vi "Roper DOE Gas Volume Consumed.vi"() -> ()   [LabVIEW 2012]
uses:
  <vilib>/DAQmx/read.llb/DAQmx Read (Analog 1D DBL NChan 1Samp).vi
  <vilib>/DAQmx/miscellaneous.llb/DAQmx Fill In Error Info.vi
panel:
  out "LP":bool
  out "NG":bool
  out "25%Sum":dbl
  out "MaxRateSum":dbl
  out "25%RateTime":dbl
  out "MaxRateTime":dbl
  out "CurrentState":string
  in  "Data Sampling Rate (s)":dbl=1.0
  out "Second":dbl format="%#.0f"
  out "Minute":dbl format="%#.0f"
  out "25PercentInRange":bool
  out "25PercentRate":bool
  out "MaxRateState":bool
  out "25% Rate Run Average":dbl format="%#.0f"
  out "Target 25% Average":dbl format="%#.0f"
  out "Max Rate Run Avg.":dbl format="%#.0f"
  out "HV":dbl
  out "CF HR":dbl
  out "Meter SLPM":dbl
  out "Sum Time":dbl
  in  "Gas Type":string
  out "Current Meter":dbl
  in  "Reset":bool
  out "Seconds":dbl format="%#.0f"
  out "Minutes":dbl format="%#.0f"
  out "Cubic Ft. Flowed":dbl format="%#.3f"
  out "Signal 2":bool
  out "Reference6":dbl
  out "Reference5":dbl
  out "Reference4":dbl
  out "Reference3":dbl
  out "Reference2":dbl
  out "Reference1":dbl
  in  "HeatingValueLP":dbl=2450.0 min=2400.0 max=2600.0 step=1.0
  out "Output 6":dbl min=0.0 max=5.0 step=0.01
  out "Output 5":dbl min=0.0 max=5.0 step=0.01
  out "Output 4":dbl min=0.0 max=5.0 step=0.01
  out "Output 3":dbl min=0.0 max=5.0 step=0.01
  out "Output 2":dbl min=0.0 max=5.0 step=0.01
  out "Output 1":dbl min=0.0 max=5.0 step=0.01
  in  "HeatingValueNG":dbl=990.0 min=950.0 max=1050.0 step=1.0
  out "Flow Rate":dbl format="%#.0f"
  # "Instant Flow Rate (BTU/hr)"
  # "Signal"
  # "Dry Heating Value"
  # "Elapsed Time"
  # ":"
  # "In Range"
  # "25% Rate Countdown Timer"
  # ":"
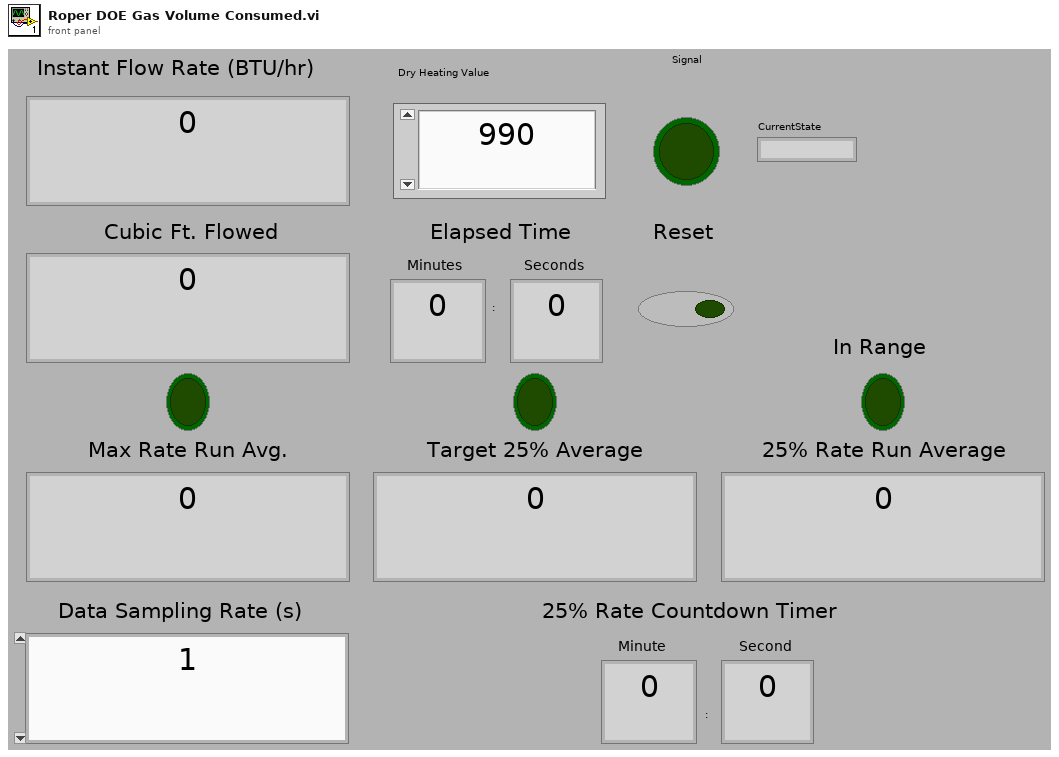
[diagram p1: front panel]
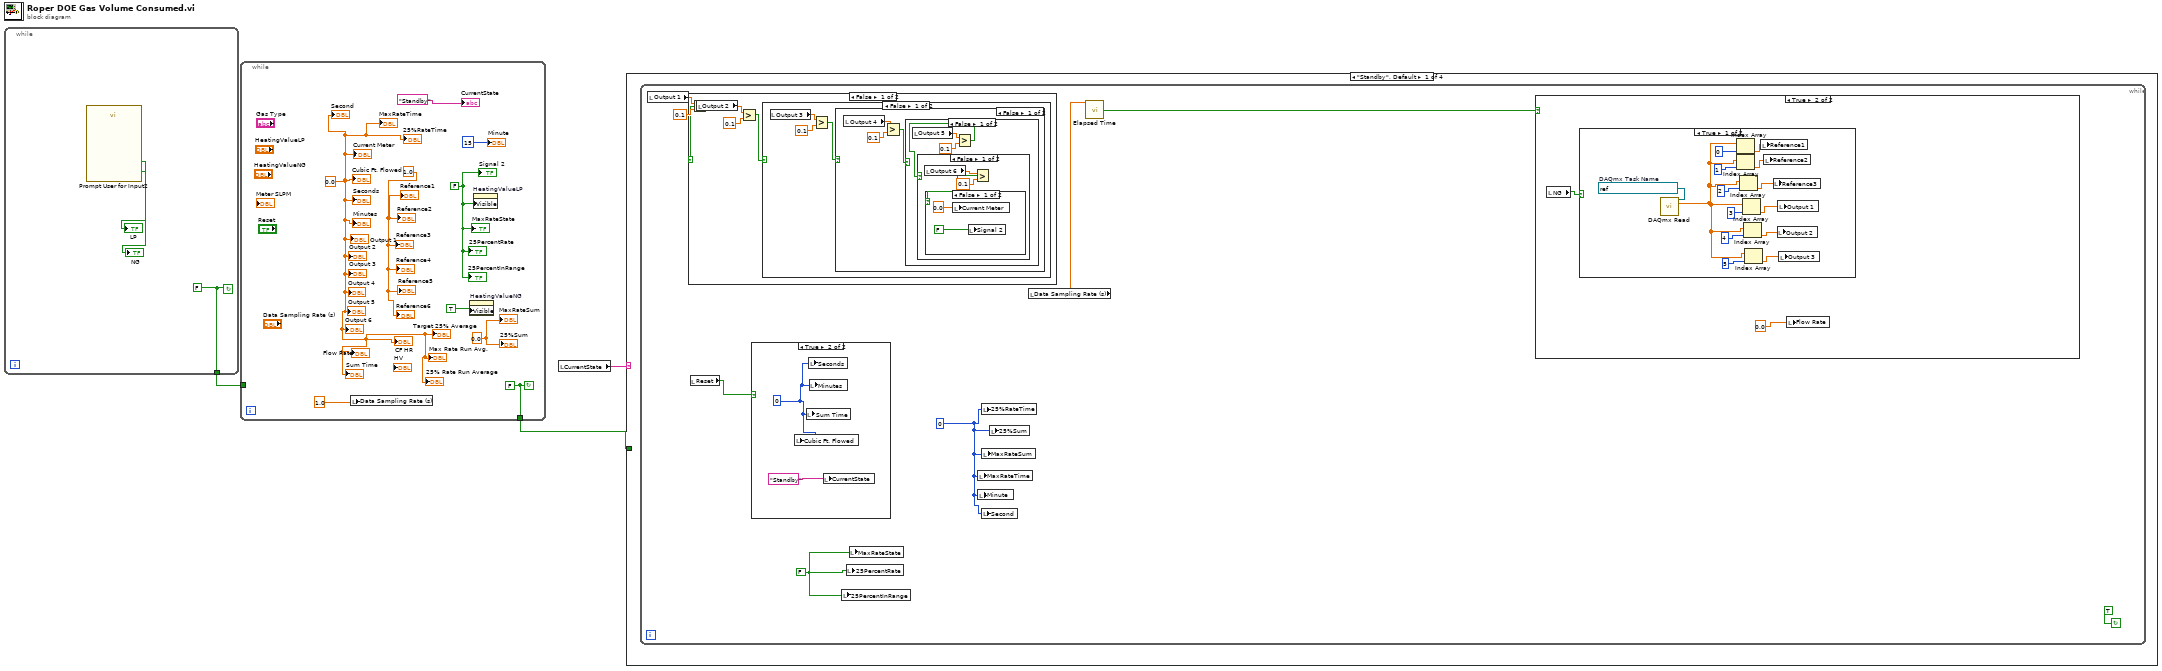
[diagram p0: block diagram]
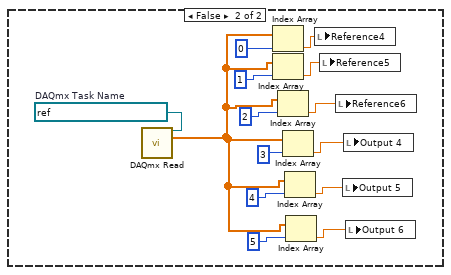
[diagram p3: hidden frame]
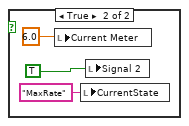
[diagram p4: hidden frame]
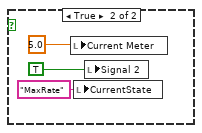
[diagram p5: hidden frame]
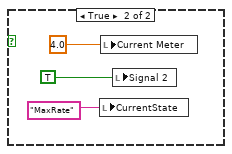
[diagram p6: hidden frame]
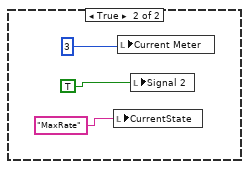
[diagram p7: hidden frame]
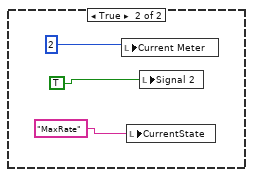
[diagram p8: hidden frame]
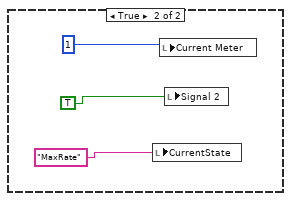
[diagram p9: hidden frame]
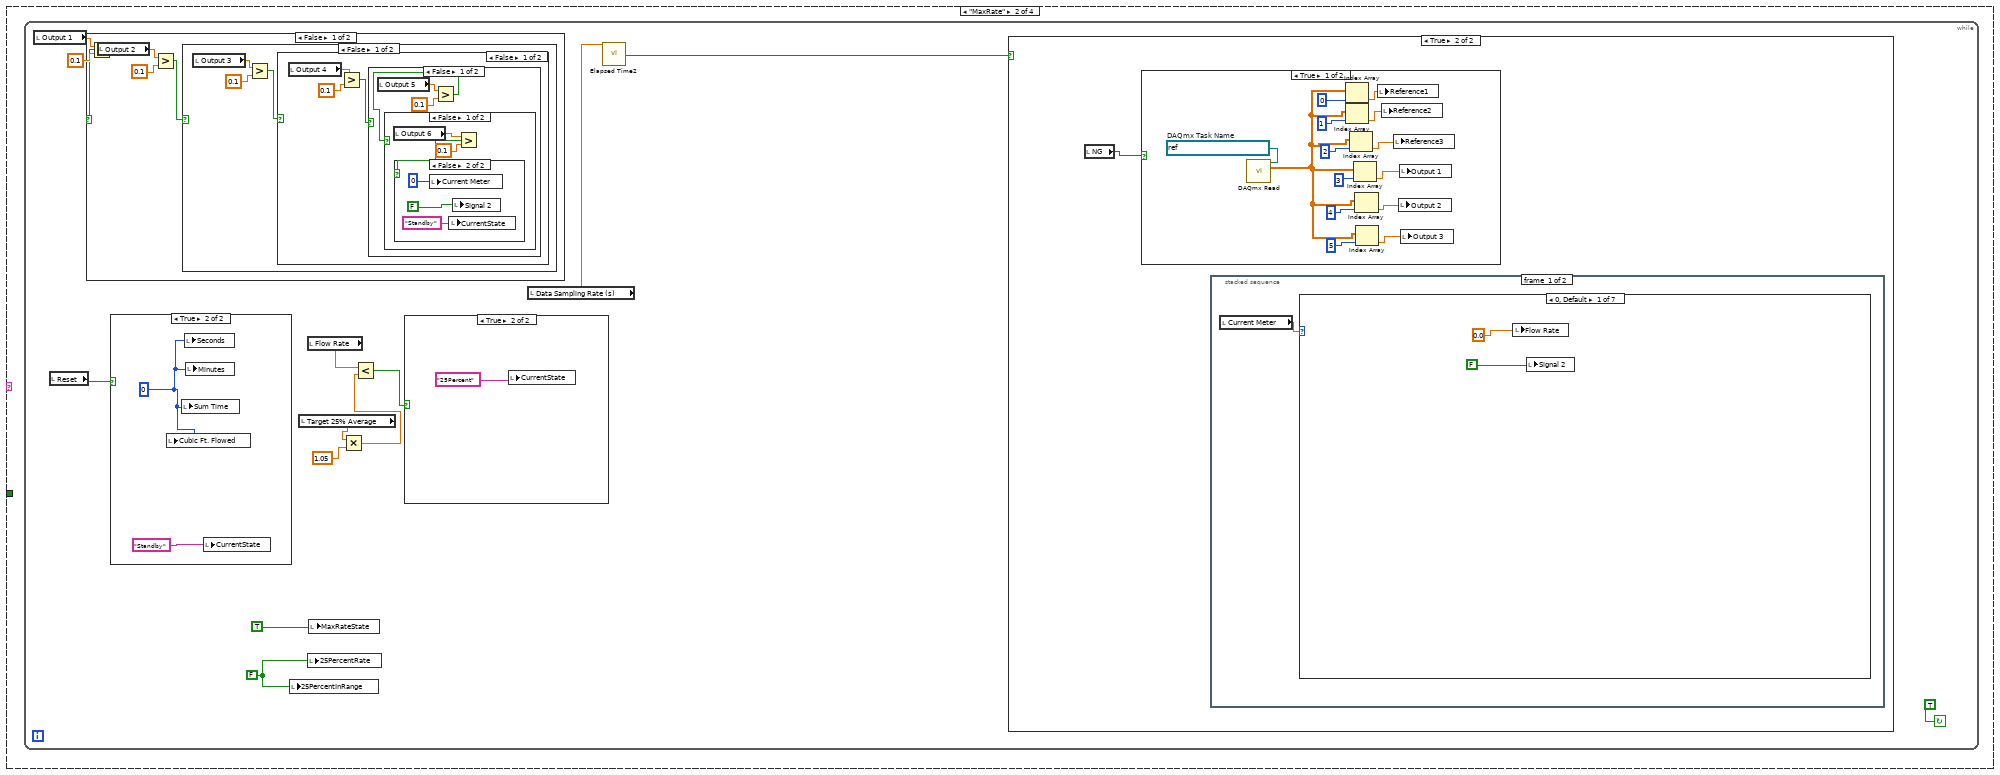
[diagram p11: hidden frame]
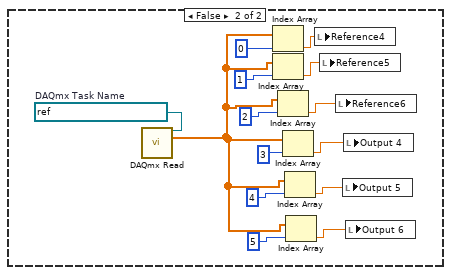
[diagram p14: hidden frame]
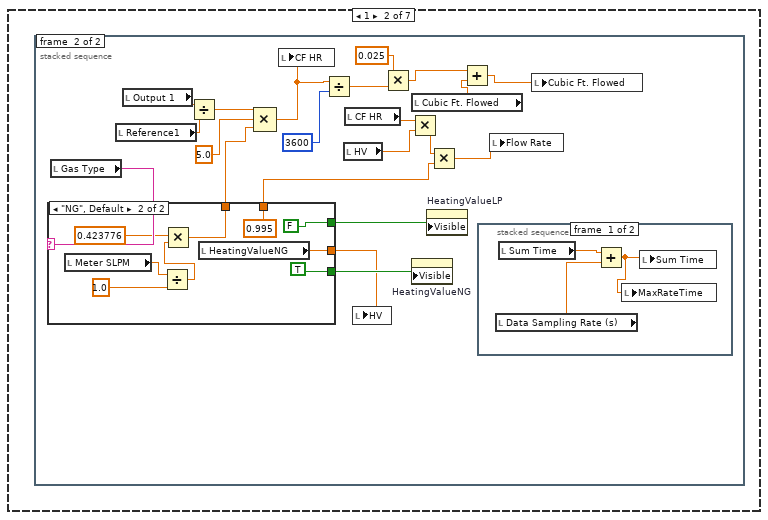
[diagram p15: hidden frame]
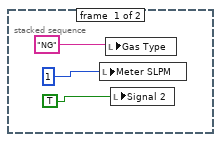
[diagram p16: hidden frame]
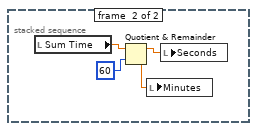
[diagram p17: hidden frame]
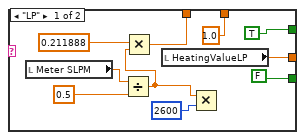
[diagram p18: hidden frame]
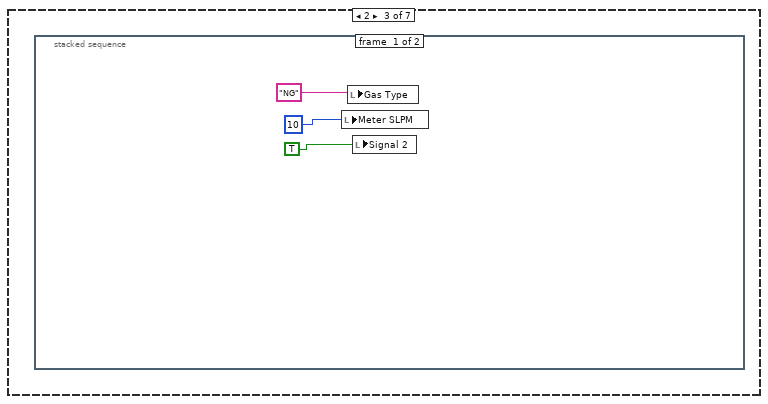
[diagram p19: hidden frame]
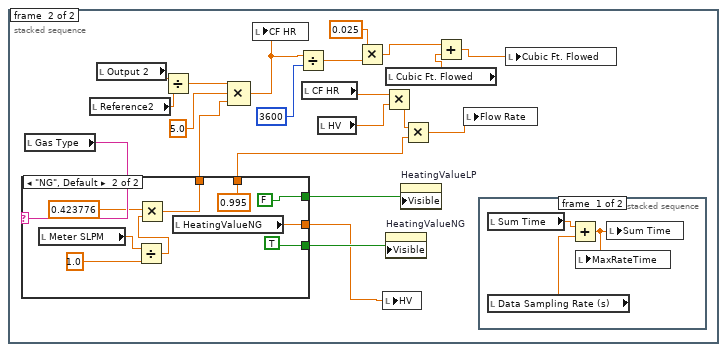
[diagram p20: hidden frame]
diagram:
  n1 = while {
    tunnel: [w6] -> w2
    stop <- w6 continue-if-true
    w6 = FALSE
    n2 = call "Prompt User for Input2"() -> ("LP"=→"LP":bool, "NG"=→"NG":bool)  [unwired: 16 in, 2 out]
  }
  n3 = while {
    tunnel: w2 -> [_]
    tunnel: [w9] -> w1
    stop <- w9 continue-if-true
    w10 = 0.0
    w13 = FALSE
    w15 = 1.0
    w8 = 0.0
    w9 = FALSE
    n4 = local write "Data Sampling Rate (s)"(1.0) -> ()
    n5 = property on="HeatingValueNG" class="DigNum (strict)"("Visible"=TRUE) -> ()  [unwired: 2 in, 2 out]
    n6 = property on="HeatingValueLP" class="DigNum (strict)"("Visible"=w13) -> ()  [unwired: 2 in, 2 out]
    "Output 1" <- w8
    "Output 2" <- w8
    "Output 3" <- w8
    "Output 4" <- w8
    "Output 5" <- w8
    "Output 6" <- w8
    "Reference1" <- w15
    "Reference2" <- w15
    "Reference3" <- w15
    "Reference4" <- w15
    "Reference5" <- w15
    "Reference6" <- w15
    "Flow Rate" <- w8
    "Signal 2" <- w13
    "Cubic Ft. Flowed" <- w8
    "Minutes" <- w8
    "Seconds" <- w8
    "Current Meter" <- w8
    "Sum Time" <- w8
    "CF HR" <- w8
    "Max Rate Run Avg." <- w8
    "Target 25% Average" <- w8
    "25% Rate Run Average" <- w8
    "MaxRateState" <- w13
    "25PercentRate" <- w13
    "25PercentInRange" <- w13
    "Minute" <- 15
    "Second" <- w8
    "CurrentState" <- "Standby"
    "25%RateTime" <- w8
    "MaxRateTime" <- w8
    "25%Sum" <- w10
    "MaxRateSum" <- w10
  }
  n7 = local read "CurrentState"() -> (w3:string)
  n8 = case shown="\"Standby\", Default" w3 {
    tunnel: w1 -> [_ _ _ _]
    frame "Standby", Default {
      n9 = while {
        stop <- TRUE continue-if-true
        w16 = 0
        w17 = FALSE
        n10 = local read "Output 1"() -> (w21:dbl)
        n11 = local read "Reset"() -> (w23:bool)
        n12 = Greater?(x=w21, y=0.1) -> (0:w20:bool)
        n13 = case shown="False" w20 {
          frame False {
            n14 = local read "Output 2"() -> (w56:dbl)
            n15 = Greater?(x=w56, y=0.1) -> (0:w55:bool)
            n16 = case shown="False" w55 {
              frame False {
                n17 = local read "Output 3"() -> (w59:dbl)
                n18 = Greater?(x=w59, y=0.1) -> (0:w58:bool)
                n19 = case shown="False" w58 {
                  frame False {
                    n20 = local read "Output 4"() -> (w63:dbl)
                    n21 = Greater?(x=w63, y=0.1) -> (0:w61:bool)
                    n22 = case shown="False" w61 {
                      frame False {
                        n23 = local read "Output 5"() -> (w66:dbl)
                        n24 = Greater?(x=w66, y=0.1) -> (0:w64:bool)
                        n25 = case shown="False" w64 {
                          frame False {
                            n26 = local read "Output 6"() -> (w68:dbl)
                            n27 = Greater?(x=w68, y=0.1) -> (0:w67:bool)
                            n28 = case shown="False" w67 {
                              frame False {
                                n29 = local write "Current Meter"(0.0) -> ()
                                n30 = local write "Signal 2"(FALSE) -> ()
                              }
                              frame True {
                                n31 = local write "Current Meter"(6.0) -> ()
                                n32 = local write "CurrentState"("MaxRate") -> ()
                                n33 = local write "Signal 2"(TRUE) -> ()
                              }
                            }
                          }
                          frame True {
                            n34 = local write "Current Meter"(5.0) -> ()
                            n35 = local write "CurrentState"("MaxRate") -> ()
                            n36 = local write "Signal 2"(TRUE) -> ()
                          }
                        }
                      }
                      frame True {
                        n37 = local write "CurrentState"("MaxRate") -> ()
                        n38 = local write "Current Meter"(4.0) -> ()
                        n39 = local write "Signal 2"(TRUE) -> ()
                      }
                    }
                  }
                  frame True {
                    n40 = local write "CurrentState"("MaxRate") -> ()
                    n41 = local write "Current Meter"(3) -> ()
                    n42 = local write "Signal 2"(TRUE) -> ()
                  }
                }
              }
              frame True {
                n43 = local write "Current Meter"(2) -> ()
                n44 = local write "CurrentState"("MaxRate") -> ()
                n45 = local write "Signal 2"(TRUE) -> ()
              }
            }
          }
          frame True {
            n46 = local write "CurrentState"("MaxRate") -> ()
            n47 = local write "Current Meter"(1) -> ()
            n48 = local write "Signal 2"(TRUE) -> ()
          }
        }
        n49 = case shown="True" w23 {
          frame False {
          }
          frame True {
            w91 = 0
            n50 = local write "Cubic Ft. Flowed"(w91) -> ()
            n51 = local write "Sum Time"(w91) -> ()
            n52 = local write "Seconds"(w91) -> ()
            n53 = local write "Minutes"(w91) -> ()
            n54 = local write "CurrentState"("Standby") -> ()
          }
        }
        n55 = local write "25PercentInRange"(w17) -> ()
        n56 = local write "25PercentRate"(w17) -> ()
        n57 = local write "MaxRateState"(w17) -> ()
        n58 = local write "MaxRateTime"(w16) -> ()
        n59 = local write "Minute"(w16) -> ()
        n60 = local write "25%RateTime"(w16) -> ()
        n61 = local write "Second"(w16) -> ()
        n62 = local write "MaxRateSum"(w16) -> ()
        n63 = local write "25%Sum"(w16) -> ()
        n64 = local read "Data Sampling Rate (s)"() -> (w18:dbl)
        n65 = call "Elapsed Time"("Time Target (s)"=w18) -> ("Time has Elapsed"=w19:bool)  [unwired: 11 in, 7 out]
        n66 = case shown="True" w19 {
          frame False {
          }
          frame True {
            n67 = local read "NG"() -> (w25:bool)
            n68 = case shown="True" w25 {
              frame True {
                w40 = refnum<k21> "ReadNGFlowMeterIn"  # DAQmx Task Name
                n69 = call-poly <vilib>:"DAQmx Read.vi"("task/channels in"=w40) -> ("data"=w31:dbl[])  [unwired: 12 in, 2 out]
                n70 = Index Array(array=w31, index=0) -> (element=w36:dbl)
                n71 = Index Array(array=w31, index=1) -> (element=w37:dbl)
                n72 = Index Array(array=w31, index=2) -> (element=w30:dbl)
                n73 = Index Array(array=w31, index=3) -> (element=w29:dbl)
                n74 = Index Array(array=w31, index=4) -> (element=w28:dbl)
                n75 = Index Array(array=w31, index=5) -> (element=w27:dbl)
                n76 = local write "Reference1"(w36) -> ()
                n77 = local write "Reference2"(w37) -> ()
                n78 = local write "Reference3"(w30) -> ()
                n79 = local write "Output 2"(w28) -> ()
                n80 = local write "Output 1"(w29) -> ()
                n81 = local write "Output 3"(w27) -> ()
              }
              frame False {
                w54 = refnum<k21> "ReadLPFlowMeterIn"  # DAQmx Task Name
                n82 = call-poly <vilib>:"DAQmx Read.vi"("task/channels in"=w54) -> ("data"=w45:dbl[])  [unwired: 12 in, 2 out]
                n83 = Index Array(array=w45, index=0) -> (element=w50:dbl)
                n84 = Index Array(array=w45, index=1) -> (element=w51:dbl)
                n85 = Index Array(array=w45, index=2) -> (element=w44:dbl)
                n86 = Index Array(array=w45, index=3) -> (element=w43:dbl)
                n87 = Index Array(array=w45, index=4) -> (element=w42:dbl)
                n88 = Index Array(array=w45, index=5) -> (element=w41:dbl)
                n89 = local write "Reference4"(w50) -> ()
                n90 = local write "Reference5"(w51) -> ()
                n91 = local write "Reference6"(w44) -> ()
                n92 = local write "Output 5"(w42) -> ()
                n93 = local write "Output 4"(w43) -> ()
                n94 = local write "Output 6"(w41) -> ()
              }
            }
            n95 = local write "Flow Rate"(0.0) -> ()
          }
        }
      }
    }
    frame "MaxRate" {
      n96 = while {
        stop <- TRUE continue-if-true
        w97 = FALSE
        n97 = local read "Output 1"() -> (w102:dbl)
        n98 = local read "Reset"() -> (w104:bool)
        n99 = Greater?(x=w102, y=0.1) -> (0:w101:bool)
        n100 = case shown="False" w101 {
          frame False {
            n101 = local read "Output 2"() -> (w451:dbl)
            n102 = Greater?(x=w451, y=0.1) -> (0:w450:bool)
            n103 = case shown="False" w450 {
              frame False {
                n104 = local read "Output 3"() -> (w454:dbl)
                n105 = Greater?(x=w454, y=0.1) -> (0:w453:bool)
                n106 = case shown="False" w453 {
                  frame False {
                    n107 = local read "Output 4"() -> (w458:dbl)
                    n108 = Greater?(x=w458, y=0.1) -> (0:w456:bool)
                    n109 = case shown="False" w456 {
                      frame False {
                        n110 = local read "Output 5"() -> (w461:dbl)
                        n111 = Greater?(x=w461, y=0.1) -> (0:w459:bool)
                        n112 = case shown="False" w459 {
                          frame False {
                            n113 = local read "Output 6"() -> (w463:dbl)
                            n114 = Greater?(x=w463, y=0.1) -> (0:w462:bool)
                            n115 = case shown="False" w462 {
                              frame True {
                                n116 = local write "Current Meter"(6.0) -> ()
                                n117 = local write "Signal 2"(TRUE) -> ()
                              }
                              frame False {
                                n118 = local write "Current Meter"(0) -> ()
                                n119 = local write "CurrentState"("Standby") -> ()
                                n120 = local write "Signal 2"(FALSE) -> ()
                              }
                            }
                          }
                          frame True {
                            n121 = local write "Current Meter"(5.0) -> ()
                            n122 = local write "Signal 2"(TRUE) -> ()
                          }
                        }
                      }
                      frame True {
                        n123 = local write "Current Meter"(4.0) -> ()
                        n124 = local write "Signal 2"(TRUE) -> ()
                      }
                    }
                  }
                  frame True {
                    n125 = local write "Current Meter"(3) -> ()
                    n126 = local write "Signal 2"(TRUE) -> ()
                  }
                }
              }
              frame True {
                n127 = local write "Current Meter"(2) -> ()
                n128 = local write "Signal 2"(TRUE) -> ()
              }
            }
          }
          frame True {
            n129 = local write "Current Meter"(1) -> ()
            n130 = local write "Signal 2"(TRUE) -> ()
          }
        }
        n131 = case shown="True" w104 {
          frame False {
          }
          frame True {
            w481 = 0
            n132 = local write "Cubic Ft. Flowed"(w481) -> ()
            n133 = local write "Sum Time"(w481) -> ()
            n134 = local write "Seconds"(w481) -> ()
            n135 = local write "Minutes"(w481) -> ()
            n136 = local write "CurrentState"("Standby") -> ()
          }
        }
        n137 = local write "25PercentInRange"(w97) -> ()
        n138 = local read "Target 25% Average"() -> (w94:dbl)
        n139 = local read "Flow Rate"() -> (w96:dbl)
        n140 = local write "25PercentRate"(w97) -> ()
        n141 = local write "MaxRateState"(TRUE) -> ()
        n142 = Multiply(x=w94, y=1.05) -> (x*y=w93:dbl)
        n143 = Less?(x=w96, y=w93) -> (x < y?=w92:bool)
        n144 = case shown="True" w92 {
          frame False {
          }
          frame True {
            n145 = local write "CurrentState"("25Percent") -> ()
          }
        }
        n146 = local read "Data Sampling Rate (s)"() -> (w99:dbl)
        n147 = call "Elapsed Time2"("Time Target (s)"=w99) -> ("Time has Elapsed"=w100:bool)  [unwired: 11 in, 7 out]
        n148 = case shown="True" w100 {
          frame False {
          }
          frame True {
            n149 = local read "NG"() -> (w107:bool)
            n150 = case shown="True" w107 {
              frame True {
                w121 = refnum<k21> "ReadNGFlowMeterIn"  # DAQmx Task Name
                n151 = call-poly <vilib>:"DAQmx Read.vi"("task/channels in"=w121) -> ("data"=w112:dbl[])  [unwired: 12 in, 2 out]
                n152 = Index Array(array=w112, index=0) -> (element=w117:dbl)
                n153 = Index Array(array=w112, index=1) -> (element=w118:dbl)
                n154 = Index Array(array=w112, index=2) -> (element=w111:dbl)
                n155 = Index Array(array=w112, index=3) -> (element=w110:dbl)
                n156 = Index Array(array=w112, index=4) -> (element=w109:dbl)
                n157 = Index Array(array=w112, index=5) -> (element=w108:dbl)
                n158 = local write "Reference1"(w117) -> ()
                n159 = local write "Reference2"(w118) -> ()
                n160 = local write "Reference3"(w111) -> ()
                n161 = local write "Output 2"(w109) -> ()
                n162 = local write "Output 1"(w110) -> ()
                n163 = local write "Output 3"(w108) -> ()
              }
              frame False {
                w135 = refnum<k21> "ReadLPFlowMeterIn"  # DAQmx Task Name
                n164 = call-poly <vilib>:"DAQmx Read.vi"("task/channels in"=w135) -> ("data"=w126:dbl[])  [unwired: 12 in, 2 out]
                n165 = Index Array(array=w126, index=0) -> (element=w131:dbl)
                n166 = Index Array(array=w126, index=1) -> (element=w132:dbl)
                n167 = Index Array(array=w126, index=2) -> (element=w125:dbl)
                n168 = Index Array(array=w126, index=3) -> (element=w124:dbl)
                n169 = Index Array(array=w126, index=4) -> (element=w123:dbl)
                n170 = Index Array(array=w126, index=5) -> (element=w122:dbl)
                n171 = local write "Reference4"(w131) -> ()
                n172 = local write "Reference5"(w132) -> ()
                n173 = local write "Reference6"(w125) -> ()
                n174 = local write "Output 5"(w123) -> ()
                n175 = local write "Output 4"(w124) -> ()
                n176 = local write "Output 6"(w122) -> ()
              }
            }
            n177 = stacked-sequence {
              frame #0 {
                n178 = local read "Current Meter"() -> (w136:dbl)
                n179 = case shown="0, Default" w136 {
                  frame 0, Default {
                    n180 = local write "Flow Rate"(0.0) -> ()
                    n181 = local write "Signal 2"(FALSE) -> ()
                  }
                  frame 1 {
                    n182 = stacked-sequence {
                      frame #0 {
                        n183 = local write "Meter SLPM"(1) -> ()
                        n184 = local write "Gas Type"("NG") -> ()
                        n185 = local write "Signal 2"(TRUE) -> ()
                      }
                      frame #1 {
                        n186 = local read "Gas Type"() -> (w154:string)
                        n187 = case shown="\"NG\", Default" w154 {
                          tunnel: [w176 w185] -> w153
                          tunnel: [TRUE FALSE] -> w152
                          tunnel: [FALSE TRUE] -> w151
                          tunnel: [1.0 0.995] -> w150
                          tunnel: [w170 w180] -> w149
                          frame "LP" {
                            n188 = local read "Meter SLPM"() -> (w178:dbl)
                            n189 = Divide(x=w178, y=0.5) -> (x/y=w171:dbl)
                            n190 = Multiply(x=0.211888, y=w171) -> (x*y=w176:dbl)
                            n191 = local read "HeatingValueLP"() -> (w170:dbl)
                            n192 = Multiply(x=w171, y=2600) -> ()  [unwired: 1 out]
                          }
                          frame "NG", Default {
                            n193 = local read "Meter SLPM"() -> (w187:dbl)
                            n194 = Divide(x=w187, y=1.0) -> (x/y=w181:dbl)
                            n195 = Multiply(x=0.423776, y=w181) -> (x*y=w185:dbl)
                            n196 = local read "HeatingValueNG"() -> (w180:dbl)
                          }
                        }
                        n197 = local read "Reference1"() -> (w157:dbl)
                        n198 = local read "Output 1"() -> (w158:dbl)
                        n199 = Divide(x=w158, y=w157) -> (x/y=w155:dbl)
                        n200 = Compound Arithmetic op=MULTIPLY(w155, 5.0, w153) -> (w148:dbl)
                        n201 = local write "CF HR"(w148) -> ()
                        n202 = Divide(x=w148, y=3600) -> (x/y=w146:dbl)
                        n203 = local read "HV"() -> (w160:dbl)
                        n204 = local read "CF HR"() -> (w159:dbl)
                        n205 = local write "HV"(w149) -> ()
                        n206 = Multiply(x=0.025, y=w146) -> (x*y=w143:dbl)
                        n207 = Multiply(x=w159, y=w160) -> (x*y=w161:dbl)
                        n208 = local read "Cubic Ft. Flowed"() -> (w144:dbl)
                        n209 = property on="HeatingValueNG" class="DigNum (strict)"("Visible"=w151) -> ()  [unwired: 2 in, 2 out]
                        n210 = property on="HeatingValueLP" class="DigNum (strict)"("Visible"=w152) -> ()  [unwired: 2 in, 2 out]
                        n211 = Multiply(x=w161, y=w150) -> (x*y=w162:dbl)
                        n212 = Add(x=w143, y=w144) -> (x+y=w142:dbl)
                        n213 = stacked-sequence {
                          frame #0 {
                            n214 = local read "Data Sampling Rate (s)"() -> (w164:dbl)
                            n215 = local read "Sum Time"() -> (w165:dbl)
                            n216 = Add(x=w165, y=w164) -> (x+y=w163:dbl)
                            n217 = local write "MaxRateTime"(w163) -> ()
                            n218 = local write "Sum Time"(w163) -> ()
                          }
                          frame #1 {
                            n219 = local read "Sum Time"() -> (w169:dbl)
                            n220 = Quotient & Remainder(x=w169, y=60) -> (x-y*floor(x/y)=w166:dbl, floor(x/y)=w167:dbl)
                            n221 = local write "Minutes"(w167) -> ()
                            n222 = local write "Seconds"(w166) -> ()
                          }
                        }
                        n223 = local write "Flow Rate"(w162) -> ()
                        n224 = local write "Cubic Ft. Flowed"(w142) -> ()
                      }
                    }
                  }
                  frame 2 {
                    n225 = stacked-sequence {
                      frame #0 {
                        n226 = local write "Meter SLPM"(10) -> ()
                        n227 = local write "Gas Type"("NG") -> ()
                        n228 = local write "Signal 2"(TRUE) -> ()
                      }
                      frame #1 {
                        n229 = local read "Gas Type"() -> (w204:string)
                        n230 = case shown="\"NG\", Default" w204 {
                          tunnel: [w226 w235] -> w203
                          tunnel: [TRUE FALSE] -> w202
                          tunnel: [FALSE TRUE] -> w201
                          tunnel: [1.0 0.995] -> w200
                          tunnel: [w220 w230] -> w199
                          frame "LP" {
                            n231 = local read "Meter SLPM"() -> (w228:dbl)
                            n232 = Divide(x=w228, y=0.5) -> (x/y=w221:dbl)
                            n233 = Multiply(x=0.211888, y=w221) -> (x*y=w226:dbl)
                            n234 = local read "HeatingValueLP"() -> (w220:dbl)
                            n235 = Multiply(x=w221, y=2600) -> ()  [unwired: 1 out]
                          }
                          frame "NG", Default {
                            n236 = local read "Meter SLPM"() -> (w237:dbl)
                            n237 = Divide(x=w237, y=1.0) -> (x/y=w231:dbl)
                            n238 = Multiply(x=0.423776, y=w231) -> (x*y=w235:dbl)
                            n239 = local read "HeatingValueNG"() -> (w230:dbl)
                          }
                        }
                        n240 = local read "Reference2"() -> (w207:dbl)
                        n241 = local read "Output 2"() -> (w208:dbl)
                        n242 = Divide(x=w208, y=w207) -> (x/y=w205:dbl)
                        n243 = Compound Arithmetic op=MULTIPLY(w205, 5.0, w203) -> (w198:dbl)
                        n244 = local write "CF HR"(w198) -> ()
                        n245 = Divide(x=w198, y=3600) -> (x/y=w196:dbl)
                        n246 = local read "CF HR"() -> (w209:dbl)
                        n247 = local read "HV"() -> (w210:dbl)
                        n248 = Multiply(x=0.025, y=w196) -> (x*y=w193:dbl)
                        n249 = local write "HV"(w199) -> ()
                        n250 = Multiply(x=w209, y=w210) -> (x*y=w211:dbl)
                        n251 = local read "Cubic Ft. Flowed"() -> (w194:dbl)
                        n252 = property on="HeatingValueNG" class="DigNum (strict)"("Visible"=w201) -> ()  [unwired: 2 in, 2 out]
                        n253 = property on="HeatingValueLP" class="DigNum (strict)"("Visible"=w202) -> ()  [unwired: 2 in, 2 out]
                        n254 = Multiply(x=w211, y=w200) -> (x*y=w212:dbl)
                        n255 = Add(x=w193, y=w194) -> (x+y=w192:dbl)
                        n256 = local write "Flow Rate"(w212) -> ()
                        n257 = stacked-sequence {
                          frame #0 {
                            n258 = local read "Sum Time"() -> (w215:dbl)
                            n259 = local read "Data Sampling Rate (s)"() -> (w214:dbl)
                            n260 = Add(x=w215, y=w214) -> (x+y=w213:dbl)
                            n261 = local write "MaxRateTime"(w213) -> ()
                            n262 = local write "Sum Time"(w213) -> ()
                          }
                          frame #1 {
                            n263 = local read "Sum Time"() -> (w219:dbl)
                            n264 = Quotient & Remainder(x=w219, y=60) -> (x-y*floor(x/y)=w216:dbl, floor(x/y)=w217:dbl)
                            n265 = local write "Minutes"(w217) -> ()
                            n266 = local write "Seconds"(w216) -> ()
                          }
                        }
                        n267 = local write "Cubic Ft. Flowed"(w192) -> ()
                      }
                    }
                  }
                  frame 3 {
                    n268 = stacked-sequence {
                      frame #0 {
                        n269 = local write "Meter SLPM"(50) -> ()
                        n270 = local write "Gas Type"("NG") -> ()
                        n271 = local write "Signal 2"(TRUE) -> ()
                      }
                      frame #1 {
                        n272 = local read "Gas Type"() -> (w254:string)
                        n273 = case shown="\"NG\", Default" w254 {
                          tunnel: [w276 w285] -> w253
                          tunnel: [TRUE FALSE] -> w252
                          tunnel: [FALSE TRUE] -> w251
                          tunnel: [1.0 0.995] -> w250
                          tunnel: [w270 w280] -> w249
                          frame "LP" {
                            n274 = local read "Meter SLPM"() -> (w278:dbl)
                            n275 = Divide(x=w278, y=0.5) -> (x/y=w271:dbl)
                            n276 = Multiply(x=0.211888, y=w271) -> (x*y=w276:dbl)
                            n277 = local read "HeatingValueLP"() -> (w270:dbl)
                            n278 = Multiply(x=w271, y=2600) -> ()  [unwired: 1 out]
                          }
                          frame "NG", Default {
                            n279 = local read "Meter SLPM"() -> (w287:dbl)
                            n280 = Divide(x=w287, y=1.0) -> (x/y=w281:dbl)
                            n281 = Multiply(x=0.423776, y=w281) -> (x*y=w285:dbl)
                            n282 = local read "HeatingValueNG"() -> (w280:dbl)
                          }
                        }
                        n283 = local read "Reference3"() -> (w257:dbl)
                        n284 = local read "Output 3"() -> (w258:dbl)
                        n285 = Divide(x=w258, y=w257) -> (x/y=w255:dbl)
                        n286 = Compound Arithmetic op=MULTIPLY(w255, 5.0, w253) -> (w248:dbl)
                        n287 = local write "CF HR"(w248) -> ()
                        n288 = Divide(x=w248, y=3600) -> (x/y=w246:dbl)
                        n289 = local read "CF HR"() -> (w259:dbl)
                        n290 = local read "HV"() -> (w260:dbl)
                        n291 = Multiply(x=0.025, y=w246) -> (x*y=w243:dbl)
                        n292 = local write "HV"(w249) -> ()
                        n293 = Multiply(x=w259, y=w260) -> (x*y=w261:dbl)
                        n294 = local read "Cubic Ft. Flowed"() -> (w244:dbl)
                        n295 = property on="HeatingValueNG" class="DigNum (strict)"("Visible"=w251) -> ()  [unwired: 2 in, 2 out]
                        n296 = property on="HeatingValueLP" class="DigNum (strict)"("Visible"=w252) -> ()  [unwired: 2 in, 2 out]
                        n297 = Multiply(x=w261, y=w250) -> (x*y=w262:dbl)
                        n298 = Add(x=w243, y=w244) -> (x+y=w242:dbl)
                        n299 = local write "Flow Rate"(w262) -> ()
                        n300 = stacked-sequence {
                          frame #0 {
                            n301 = local read "Data Sampling Rate (s)"() -> (w264:dbl)
                            n302 = local read "Sum Time"() -> (w265:dbl)
                            n303 = Add(x=w265, y=w264) -> (x+y=w263:dbl)
                            n304 = local write "MaxRateTime"(w263) -> ()
                            n305 = local write "Sum Time"(w263) -> ()
                          }
                          frame #1 {
                            n306 = local read "Sum Time"() -> (w269:dbl)
                            n307 = Quotient & Remainder(x=w269, y=60) -> (x-y*floor(x/y)=w266:dbl, floor(x/y)=w267:dbl)
                            n308 = local write "Minutes"(w267) -> ()
                            n309 = local write "Seconds"(w266) -> ()
                          }
                        }
                        n310 = local write "Cubic Ft. Flowed"(w242) -> ()
                      }
                    }
                  }
                  frame 4 {
                    n311 = stacked-sequence {
                      frame #0 {
                        n312 = local write "Meter SLPM"(0.5) -> ()
                        n313 = local write "Gas Type"("LP") -> ()
                        n314 = local write "Signal 2"(TRUE) -> ()
                      }
                      frame #1 {
                        n315 = local read "Gas Type"() -> (w304:string)
                        n316 = case shown="\"NG\", Default" w304 {
                          tunnel: [w326 w335] -> w303
                          tunnel: [TRUE FALSE] -> w302
                          tunnel: [FALSE TRUE] -> w301
                          tunnel: [1.0 0.995] -> w300
                          tunnel: [w320 w330] -> w299
                          frame "LP" {
                            n317 = local read "Meter SLPM"() -> (w328:dbl)
                            n318 = Divide(x=w328, y=0.5) -> (x/y=w321:dbl)
                            n319 = Multiply(x=0.211888, y=w321) -> (x*y=w326:dbl)
                            n320 = local read "HeatingValueLP"() -> (w320:dbl)
                            n321 = Multiply(x=w321, y=2600) -> ()  [unwired: 1 out]
                          }
                          frame "NG", Default {
                            n322 = local read "Meter SLPM"() -> (w337:dbl)
                            n323 = Divide(x=w337, y=1.0) -> (x/y=w331:dbl)
                            n324 = Multiply(x=0.423776, y=w331) -> (x*y=w335:dbl)
                            n325 = local read "HeatingValueNG"() -> (w330:dbl)
                          }
                        }
                        n326 = local read "Reference4"() -> (w307:dbl)
                        n327 = local read "Output 4"() -> (w308:dbl)
                        n328 = Divide(x=w308, y=w307) -> (x/y=w305:dbl)
                        n329 = Compound Arithmetic op=MULTIPLY(w305, 5.0, w303) -> (w298:dbl)
                        n330 = local write "CF HR"(w298) -> ()
                        n331 = Divide(x=w298, y=3600) -> (x/y=w296:dbl)
                        n332 = local read "CF HR"() -> (w309:dbl)
                        n333 = local read "HV"() -> (w310:dbl)
                        n334 = Multiply(x=0.025, y=w296) -> (x*y=w293:dbl)
                        n335 = local write "HV"(w299) -> ()
                        n336 = Multiply(x=w309, y=w310) -> (x*y=w311:dbl)
                        n337 = local read "Cubic Ft. Flowed"() -> (w294:dbl)
                        n338 = property on="HeatingValueNG" class="DigNum (strict)"("Visible"=w301) -> ()  [unwired: 2 in, 2 out]
                        n339 = property on="HeatingValueLP" class="DigNum (strict)"("Visible"=w302) -> ()  [unwired: 2 in, 2 out]
                        n340 = Multiply(x=w311, y=w300) -> (x*y=w312:dbl)
                        n341 = Add(x=w293, y=w294) -> (x+y=w292:dbl)
                        n342 = local write "Flow Rate"(w312) -> ()
                        n343 = stacked-sequence {
                          frame #0 {
                            n344 = local read "Sum Time"() -> (w315:dbl)
                            n345 = local read "Data Sampling Rate (s)"() -> (w314:dbl)
                            n346 = Add(x=w315, y=w314) -> (x+y=w313:dbl)
                            n347 = local write "MaxRateTime"(w313) -> ()
                            n348 = local write "Sum Time"(w313) -> ()
                          }
                          frame #1 {
                            n349 = local read "Sum Time"() -> (w319:dbl)
                            n350 = Quotient & Remainder(x=w319, y=60) -> (x-y*floor(x/y)=w316:dbl, floor(x/y)=w317:dbl)
                            n351 = local write "Minutes"(w317) -> ()
                            n352 = local write "Seconds"(w316) -> ()
                          }
                        }
                        n353 = local write "Cubic Ft. Flowed"(w292) -> ()
                      }
                    }
                  }
                  frame 5 {
                    n354 = stacked-sequence {
                      frame #0 {
                        n355 = local write "Meter SLPM"(5) -> ()
                        n356 = local write "Gas Type"("LP") -> ()
                        n357 = local write "Signal 2"(TRUE) -> ()
                      }
                      frame #1 {
                        n358 = local read "Gas Type"() -> (w354:string)
                        n359 = case shown="\"NG\", Default" w354 {
                          tunnel: [w376 w385] -> w353
                          tunnel: [TRUE FALSE] -> w352
                          tunnel: [FALSE TRUE] -> w351
                          tunnel: [1.0 0.995] -> w350
                          tunnel: [w370 w380] -> w349
                          frame "LP" {
                            n360 = local read "Meter SLPM"() -> (w378:dbl)
                            n361 = Divide(x=w378, y=0.5) -> (x/y=w371:dbl)
                            n362 = Multiply(x=0.211888, y=w371) -> (x*y=w376:dbl)
                            n363 = local read "HeatingValueLP"() -> (w370:dbl)
                            n364 = Multiply(x=w371, y=2600) -> ()  [unwired: 1 out]
                          }
                          frame "NG", Default {
                            n365 = local read "Meter SLPM"() -> (w387:dbl)
                            n366 = Divide(x=w387, y=1.0) -> (x/y=w381:dbl)
                            n367 = Multiply(x=0.423776, y=w381) -> (x*y=w385:dbl)
                            n368 = local read "HeatingValueNG"() -> (w380:dbl)
                          }
                        }
                        n369 = local read "Reference5"() -> (w357:dbl)
                        n370 = local read "Output 5"() -> (w358:dbl)
                        n371 = Divide(x=w358, y=w357) -> (x/y=w355:dbl)
                        n372 = Compound Arithmetic op=MULTIPLY(w355, 5.0, w353) -> (w348:dbl)
                        n373 = local write "CF HR"(w348) -> ()
                        n374 = Divide(x=w348, y=3600) -> (x/y=w346:dbl)
                        n375 = local read "CF HR"() -> (w359:dbl)
                        n376 = local read "HV"() -> (w360:dbl)
                        n377 = Multiply(x=0.025, y=w346) -> (x*y=w343:dbl)
                        n378 = local write "HV"(w349) -> ()
                        n379 = Multiply(x=w359, y=w360) -> (x*y=w361:dbl)
                        n380 = local read "Cubic Ft. Flowed"() -> (w344:dbl)
                        n381 = property on="HeatingValueNG" class="DigNum (strict)"("Visible"=w351) -> ()  [unwired: 2 in, 2 out]
                        n382 = property on="HeatingValueLP" class="DigNum (strict)"("Visible"=w352) -> ()  [unwired: 2 in, 2 out]
                        n383 = Multiply(x=w361, y=w350) -> (x*y=w362:dbl)
                        n384 = Add(x=w343, y=w344) -> (x+y=w342:dbl)
                        n385 = local write "Flow Rate"(w362) -> ()
                        n386 = stacked-sequence {
                          frame #0 {
                            n387 = local read "Sum Time"() -> (w365:dbl)
                            n388 = local read "Data Sampling Rate (s)"() -> (w364:dbl)
                            n389 = Add(x=w365, y=w364) -> (x+y=w363:dbl)
                            n390 = local write "MaxRateTime"(w363) -> ()
                            n391 = local write "Sum Time"(w363) -> ()
                          }
                          frame #1 {
                            n392 = local read "Sum Time"() -> (w369:dbl)
                            n393 = Quotient & Remainder(x=w369, y=60) -> (x-y*floor(x/y)=w366:dbl, floor(x/y)=w367:dbl)
                            n394 = local write "Minutes"(w367) -> ()
                            n395 = local write "Seconds"(w366) -> ()
                          }
                        }
                        n396 = local write "Cubic Ft. Flowed"(w342) -> ()
                      }
                    }
                  }
                  frame 6 {
                    n397 = stacked-sequence {
                      frame #0 {
                        n398 = local write "Meter SLPM"(20) -> ()
                        n399 = local write "Gas Type"("LP") -> ()
                        n400 = local write "Signal 2"(TRUE) -> ()
                      }
                      frame #1 {
                        n401 = local read "Gas Type"() -> (w404:string)
                        n402 = case shown="\"NG\", Default" w404 {
                          tunnel: [w426 w435] -> w403
                          tunnel: [TRUE FALSE] -> w402
                          tunnel: [FALSE TRUE] -> w401
                          tunnel: [1.0 0.995] -> w400
                          tunnel: [w420 w430] -> w399
                          frame "LP" {
                            n403 = local read "Meter SLPM"() -> (w428:dbl)
                            n404 = Divide(x=w428, y=0.5) -> (x/y=w421:dbl)
                            n405 = Multiply(x=0.211888, y=w421) -> (x*y=w426:dbl)
                            n406 = local read "HeatingValueLP"() -> (w420:dbl)
                            n407 = Multiply(x=w421, y=2600) -> ()  [unwired: 1 out]
                          }
                          frame "NG", Default {
                            n408 = local read "Meter SLPM"() -> (w437:dbl)
                            n409 = Divide(x=w437, y=1.0) -> (x/y=w431:dbl)
                            n410 = Multiply(x=0.423776, y=w431) -> (x*y=w435:dbl)
                            n411 = local read "HeatingValueNG"() -> (w430:dbl)
                          }
                        }
                        n412 = local read "Reference6"() -> (w407:dbl)
                        n413 = local read "Output 6"() -> (w408:dbl)
                        n414 = Divide(x=w408, y=w407) -> (x/y=w405:dbl)
                        n415 = Compound Arithmetic op=MULTIPLY(w405, 5.0, w403) -> (w398:dbl)
                        n416 = local write "CF HR"(w398) -> ()
                        n417 = Divide(x=w398, y=3600) -> (x/y=w396:dbl)
                        n418 = local read "CF HR"() -> (w409:dbl)
                        n419 = local read "HV"() -> (w410:dbl)
                        n420 = Multiply(x=0.025, y=w396) -> (x*y=w393:dbl)
                        n421 = local write "HV"(w399) -> ()
                        n422 = Multiply(x=w409, y=w410) -> (x*y=w411:dbl)
                        n423 = local read "Cubic Ft. Flowed"() -> (w394:dbl)
                        n424 = property on="HeatingValueNG" class="DigNum (strict)"("Visible"=w401) -> ()  [unwired: 2 in, 2 out]
                        n425 = property on="HeatingValueLP" class="DigNum (strict)"("Visible"=w402) -> ()  [unwired: 2 in, 2 out]
                        n426 = Multiply(x=w411, y=w400) -> (x*y=w412:dbl)
                        n427 = Add(x=w393, y=w394) -> (x+y=w392:dbl)
                        n428 = stacked-sequence {
                          frame #0 {
                            n429 = local read "Data Sampling Rate (s)"() -> (w414:dbl)
                            n430 = local read "Sum Time"() -> (w415:dbl)
                            n431 = Add(x=w415, y=w414) -> (x+y=w413:dbl)
                            n432 = local write "MaxRateTime"(w413) -> ()
                            n433 = local write "Sum Time"(w413) -> ()
                          }
                          frame #1 {
                            n434 = local read "Sum Time"() -> (w419:dbl)
                            n435 = Quotient & Remainder(x=w419, y=60) -> (x-y*floor(x/y)=w416:dbl, floor(x/y)=w417:dbl)
                            n436 = local write "Minutes"(w417) -> ()
                            n437 = local write "Seconds"(w416) -> ()
                          }
                        }
                        n438 = local write "Flow Rate"(w412) -> ()
                        n439 = local write "Cubic Ft. Flowed"(w392) -> ()
                      }
                    }
                  }
                }
              }
              frame #1 {
                n440 = stacked-sequence {
                  frame #0 {
                    n441 = local read "MaxRateSum"() -> (w442:dbl)
                    n442 = local read "Flow Rate"() -> (w443:dbl)
                    n443 = local read "MaxRateTime"() -> (w441:dbl)
                    n444 = Add(x=w443, y=w442) -> (x+y=w440:dbl)
                    n445 = Divide(x=w440, y=w441) -> (x/y=w439:dbl)
                    n446 = local write "Max Rate Run Avg."(w439) -> ()
                  }
                  frame #1 {
                    n447 = local read "MaxRateSum"() -> (w445:dbl)
                    n448 = local read "Flow Rate"() -> (w444:dbl)
                    n449 = Add(x=w444, y=w445) -> (x+y=w446:dbl)
                    n450 = local write "MaxRateSum"(w446) -> ()
                  }
                  frame #2 {
                    n451 = local read "Max Rate Run Avg."() -> (w449:dbl)
                    n452 = Divide(x=w449, y=4.0) -> (x/y=w447:dbl)
                    n453 = local write "Target 25% Average"(w447) -> ()
                  }
                }
              }
            }
          }
        }
      }
    }
    frame "25Percent" {
      n454 = while {
        stop <- TRUE continue-if-true
        n455 = local read "Output 1"() -> (w499:dbl)
        n456 = local read "Reset"() -> (w501:bool)
        n457 = Greater?(x=w499, y=0.1) -> (0:w498:bool)
        n458 = case shown="False" w498 {
          frame False {
            n459 = local read "Output 2"() -> (w847:dbl)
            n460 = Greater?(x=w847, y=0.1) -> (0:w846:bool)
            n461 = case shown="False" w846 {
              frame False {
                n462 = local read "Output 3"() -> (w850:dbl)
                n463 = Greater?(x=w850, y=0.1) -> (0:w849:bool)
                n464 = case shown="False" w849 {
                  frame False {
                    n465 = local read "Output 4"() -> (w854:dbl)
                    n466 = Greater?(x=w854, y=0.1) -> (0:w852:bool)
                    n467 = case shown="False" w852 {
                      frame False {
                        n468 = local read "Output 5"() -> (w857:dbl)
                        n469 = Greater?(x=w857, y=0.1) -> (0:w855:bool)
                        n470 = case shown="False" w855 {
                          frame False {
                            n471 = local read "Output 6"() -> (w859:dbl)
                            n472 = Greater?(x=w859, y=0.1) -> (0:w858:bool)
                            n473 = case shown="False" w858 {
                              frame True {
                                n474 = local write "Current Meter"(6.0) -> ()
                                n475 = local write "Signal 2"(TRUE) -> ()
                              }
                              frame False {
                                n476 = local write "Current Meter"(0) -> ()
                                n477 = local write "CurrentState"("Standby") -> ()
                                n478 = local write "Signal 2"(FALSE) -> ()
                              }
                            }
                          }
                          frame True {
                            n479 = local write "Current Meter"(5.0) -> ()
                            n480 = local write "Signal 2"(TRUE) -> ()
                          }
                        }
                      }
                      frame True {
                        n481 = local write "Current Meter"(4.0) -> ()
                        n482 = local write "Signal 2"(TRUE) -> ()
                      }
                    }
                  }
                  frame True {
                    n483 = local write "Current Meter"(3) -> ()
                    n484 = local write "Signal 2"(TRUE) -> ()
                  }
                }
              }
              frame True {
                n485 = local write "Current Meter"(2) -> ()
                n486 = local write "Signal 2"(TRUE) -> ()
              }
            }
          }
          frame True {
            n487 = local write "Current Meter"(1) -> ()
            n488 = local write "Signal 2"(TRUE) -> ()
          }
        }
        n489 = case shown="True" w501 {
          frame False {
          }
          frame True {
            w877 = 0
            n490 = local write "Cubic Ft. Flowed"(w877) -> ()
            n491 = local write "Sum Time"(w877) -> ()
            n492 = local write "Seconds"(w877) -> ()
            n493 = local write "Minutes"(w877) -> ()
            n494 = local write "CurrentState"("Standby") -> ()
          }
        }
        n495 = local read "Target 25% Average"() -> (w488:dbl)
        n496 = local read "Flow Rate"() -> (w491:dbl)
        n497 = local write "25PercentRate"(TRUE) -> ()
        n498 = local write "MaxRateState"(FALSE) -> ()
        n499 = local read "25%RateTime"() -> (w483:dbl)
        n500 = Multiply(x=w488, y=1.05) -> (x*y=w492:dbl)
        n501 = Less?(x=w491, y=w492) -> (x < y?=w486:bool)
        n502 = Greater Or Equal?(x=w483, y=900) -> (x >= y?=w482:bool)
        n503 = Multiply(x=w488, y=0.95) -> (x*y=w489:dbl)
        n504 = Greater?(x=w491, y=w489) -> (0:w487:bool)
        n505 = case shown="True" w482 {
          frame False {
          }
          frame True {
            n506 = local write "CurrentState"("Complete") -> ()
          }
        }
        n507 = And(x=w487, y=w486) -> (x .and. y?=w485:bool)
        n508 = local write "25PercentInRange"(w485) -> ()
        n509 = local read "Data Sampling Rate (s)"() -> (w496:dbl)
        n510 = call "Elapsed Time3"("Time Target (s)"=w496) -> ("Time has Elapsed"=w497:bool)  [unwired: 11 in, 7 out]
        n511 = case shown="True" w497 {
          frame False {
          }
          frame True {
            n512 = local read "NG"() -> (w504:bool)
            n513 = stacked-sequence {
              frame #0 {
                n514 = local read "Current Meter"() -> (w533:dbl)
                n515 = case shown="6" w533 {
                  frame 0, Default {
                    n516 = local write "Flow Rate"(0.0) -> ()
                    n517 = local write "Signal 2"(FALSE) -> ()
                  }
                  frame 1 {
                    n518 = stacked-sequence {
                      frame #0 {
                        n519 = local write "Meter SLPM"(1) -> ()
                        n520 = local write "Gas Type"("NG") -> ()
                        n521 = local write "Signal 2"(TRUE) -> ()
                      }
                      frame #1 {
                        n522 = local read "Gas Type"() -> (w551:string)
                        n523 = case shown="\"NG\", Default" w551 {
                          tunnel: [w573 w582] -> w550
                          tunnel: [TRUE FALSE] -> w549
                          tunnel: [FALSE TRUE] -> w548
                          tunnel: [1.0 0.995] -> w547
                          tunnel: [w567 w577] -> w546
                          frame "LP" {
                            n524 = local read "Meter SLPM"() -> (w575:dbl)
                            n525 = Divide(x=w575, y=0.5) -> (x/y=w568:dbl)
                            n526 = Multiply(x=0.211888, y=w568) -> (x*y=w573:dbl)
                            n527 = local read "HeatingValueLP"() -> (w567:dbl)
                            n528 = Multiply(x=w568, y=2600) -> ()  [unwired: 1 out]
                          }
                          frame "NG", Default {
                            n529 = local read "Meter SLPM"() -> (w584:dbl)
                            n530 = Divide(x=w584, y=1.0) -> (x/y=w578:dbl)
                            n531 = Multiply(x=0.423776, y=w578) -> (x*y=w582:dbl)
                            n532 = local read "HeatingValueNG"() -> (w577:dbl)
                          }
                        }
                        n533 = local read "Reference1"() -> (w554:dbl)
                        n534 = local read "Output 1"() -> (w555:dbl)
                        n535 = Divide(x=w555, y=w554) -> (x/y=w552:dbl)
                        n536 = Compound Arithmetic op=MULTIPLY(w552, 5.0, w550) -> (w545:dbl)
                        n537 = local write "CF HR"(w545) -> ()
                        n538 = Divide(x=w545, y=3600) -> (x/y=w543:dbl)
                        n539 = local read "HV"() -> (w557:dbl)
                        n540 = local read "CF HR"() -> (w556:dbl)
                        n541 = local write "HV"(w546) -> ()
                        n542 = Multiply(x=0.025, y=w543) -> (x*y=w540:dbl)
                        n543 = Multiply(x=w556, y=w557) -> (x*y=w558:dbl)
                        n544 = local read "Cubic Ft. Flowed"() -> (w541:dbl)
                        n545 = property on="HeatingValueNG" class="DigNum (strict)"("Visible"=w548) -> ()  [unwired: 2 in, 2 out]
                        n546 = property on="HeatingValueLP" class="DigNum (strict)"("Visible"=w549) -> ()  [unwired: 2 in, 2 out]
                        n547 = Multiply(x=w558, y=w547) -> (x*y=w559:dbl)
                        n548 = Add(x=w540, y=w541) -> (x+y=w539:dbl)
                        n549 = stacked-sequence {
                          frame #0 {
                            n550 = local read "Data Sampling Rate (s)"() -> (w561:dbl)
                            n551 = local read "Sum Time"() -> (w562:dbl)
                            n552 = Add(x=w562, y=w561) -> (x+y=w560:dbl)
                            n553 = local write "25%RateTime"(w560) -> ()
                            n554 = local write "Sum Time"(w560) -> ()
                          }
                          frame #1 {
                            n555 = local read "Sum Time"() -> (w566:dbl)
                            n556 = Quotient & Remainder(x=w566, y=60) -> (x-y*floor(x/y)=w563:dbl, floor(x/y)=w564:dbl)
                            n557 = local write "Minutes"(w564) -> ()
                            n558 = local write "Seconds"(w563) -> ()
                          }
                        }
                        n559 = local write "Flow Rate"(w559) -> ()
                        n560 = local write "Cubic Ft. Flowed"(w539) -> ()
                      }
                    }
                  }
                  frame 2 {
                    n561 = stacked-sequence {
                      frame #0 {
                        n562 = local write "Meter SLPM"(10) -> ()
                        n563 = local write "Gas Type"("NG") -> ()
                        n564 = local write "Signal 2"(TRUE) -> ()
                      }
                      frame #1 {
                        n565 = local read "Gas Type"() -> (w601:string)
                        n566 = case shown="\"NG\", Default" w601 {
                          tunnel: [w623 w632] -> w600
                          tunnel: [TRUE FALSE] -> w599
                          tunnel: [FALSE TRUE] -> w598
                          tunnel: [1.0 0.995] -> w597
                          tunnel: [w617 w627] -> w596
                          frame "LP" {
                            n567 = local read "Meter SLPM"() -> (w625:dbl)
                            n568 = Divide(x=w625, y=0.5) -> (x/y=w618:dbl)
                            n569 = Multiply(x=0.211888, y=w618) -> (x*y=w623:dbl)
                            n570 = local read "HeatingValueLP"() -> (w617:dbl)
                            n571 = Multiply(x=w618, y=2600) -> ()  [unwired: 1 out]
                          }
                          frame "NG", Default {
                            n572 = local read "Meter SLPM"() -> (w634:dbl)
                            n573 = Divide(x=w634, y=1.0) -> (x/y=w628:dbl)
                            n574 = Multiply(x=0.423776, y=w628) -> (x*y=w632:dbl)
                            n575 = local read "HeatingValueNG"() -> (w627:dbl)
                          }
                        }
                        n576 = local read "Reference2"() -> (w604:dbl)
                        n577 = local read "Output 2"() -> (w605:dbl)
                        n578 = Divide(x=w605, y=w604) -> (x/y=w602:dbl)
                        n579 = Compound Arithmetic op=MULTIPLY(w602, 5.0, w600) -> (w595:dbl)
                        n580 = local write "CF HR"(w595) -> ()
                        n581 = Divide(x=w595, y=3600) -> (x/y=w593:dbl)
                        n582 = local read "CF HR"() -> (w606:dbl)
                        n583 = local read "HV"() -> (w607:dbl)
                        n584 = Multiply(x=0.025, y=w593) -> (x*y=w590:dbl)
                        n585 = local write "HV"(w596) -> ()
                        n586 = Multiply(x=w606, y=w607) -> (x*y=w608:dbl)
                        n587 = local read "Cubic Ft. Flowed"() -> (w591:dbl)
                        n588 = property on="HeatingValueNG" class="DigNum (strict)"("Visible"=w598) -> ()  [unwired: 2 in, 2 out]
                        n589 = property on="HeatingValueLP" class="DigNum (strict)"("Visible"=w599) -> ()  [unwired: 2 in, 2 out]
                        n590 = Multiply(x=w608, y=w597) -> (x*y=w609:dbl)
                        n591 = Add(x=w590, y=w591) -> (x+y=w589:dbl)
                        n592 = local write "Flow Rate"(w609) -> ()
                        n593 = stacked-sequence {
                          frame #0 {
                            n594 = local read "Sum Time"() -> (w612:dbl)
                            n595 = local read "Data Sampling Rate (s)"() -> (w611:dbl)
                            n596 = Add(x=w612, y=w611) -> (x+y=w610:dbl)
                            n597 = local write "25%RateTime"(w610) -> ()
                            n598 = local write "Sum Time"(w610) -> ()
                          }
                          frame #1 {
                            n599 = local read "Sum Time"() -> (w616:dbl)
                            n600 = Quotient & Remainder(x=w616, y=60) -> (x-y*floor(x/y)=w613:dbl, floor(x/y)=w614:dbl)
                            n601 = local write "Minutes"(w614) -> ()
                            n602 = local write "Seconds"(w613) -> ()
                          }
                        }
                        n603 = local write "Cubic Ft. Flowed"(w589) -> ()
                      }
                    }
                  }
                  frame 3 {
                    n604 = stacked-sequence {
                      frame #0 {
                        n605 = local write "Meter SLPM"(20) -> ()
                        n606 = local write "Gas Type"("NG") -> ()
                        n607 = local write "Signal 2"(TRUE) -> ()
                      }
                      frame #1 {
                        n608 = local read "Gas Type"() -> (w651:string)
                        n609 = case shown="\"NG\", Default" w651 {
                          tunnel: [w673 w682] -> w650
                          tunnel: [TRUE FALSE] -> w649
                          tunnel: [FALSE TRUE] -> w648
                          tunnel: [1.0 0.995] -> w647
                          tunnel: [w667 w677] -> w646
                          frame "LP" {
                            n610 = local read "Meter SLPM"() -> (w675:dbl)
                            n611 = Divide(x=w675, y=0.5) -> (x/y=w668:dbl)
                            n612 = Multiply(x=0.211888, y=w668) -> (x*y=w673:dbl)
                            n613 = local read "HeatingValueLP"() -> (w667:dbl)
                            n614 = Multiply(x=w668, y=2600) -> ()  [unwired: 1 out]
                          }
                          frame "NG", Default {
                            n615 = local read "Meter SLPM"() -> (w684:dbl)
                            n616 = Divide(x=w684, y=1.0) -> (x/y=w678:dbl)
                            n617 = Multiply(x=0.423776, y=w678) -> (x*y=w682:dbl)
                            n618 = local read "HeatingValueNG"() -> (w677:dbl)
                          }
                        }
                        n619 = local read "Reference3"() -> (w654:dbl)
                        n620 = local read "Output 3"() -> (w655:dbl)
                        n621 = Divide(x=w655, y=w654) -> (x/y=w652:dbl)
                        n622 = Compound Arithmetic op=MULTIPLY(w652, 5.0, w650) -> (w645:dbl)
                        n623 = local write "CF HR"(w645) -> ()
                        n624 = Divide(x=w645, y=3600) -> (x/y=w643:dbl)
                        n625 = local read "CF HR"() -> (w656:dbl)
                        n626 = local read "HV"() -> (w657:dbl)
                        n627 = Multiply(x=0.025, y=w643) -> (x*y=w640:dbl)
                        n628 = local write "HV"(w646) -> ()
                        n629 = Multiply(x=w656, y=w657) -> (x*y=w658:dbl)
                        n630 = local read "Cubic Ft. Flowed"() -> (w641:dbl)
                        n631 = property on="HeatingValueNG" class="DigNum (strict)"("Visible"=w648) -> ()  [unwired: 2 in, 2 out]
                        n632 = property on="HeatingValueLP" class="DigNum (strict)"("Visible"=w649) -> ()  [unwired: 2 in, 2 out]
                        n633 = Multiply(x=w658, y=w647) -> (x*y=w659:dbl)
                        n634 = Add(x=w640, y=w641) -> (x+y=w639:dbl)
                        n635 = local write "Flow Rate"(w659) -> ()
                        n636 = stacked-sequence {
                          frame #0 {
                            n637 = local read "Data Sampling Rate (s)"() -> (w661:dbl)
                            n638 = local read "Sum Time"() -> (w662:dbl)
                            n639 = Add(x=w662, y=w661) -> (x+y=w660:dbl)
                            n640 = local write "25%RateTime"(w660) -> ()
                            n641 = local write "Sum Time"(w660) -> ()
                          }
                          frame #1 {
                            n642 = local read "Sum Time"() -> (w666:dbl)
                            n643 = Quotient & Remainder(x=w666, y=60) -> (x-y*floor(x/y)=w663:dbl, floor(x/y)=w664:dbl)
                            n644 = local write "Minutes"(w664) -> ()
                            n645 = local write "Seconds"(w663) -> ()
                          }
                        }
                        n646 = local write "Cubic Ft. Flowed"(w639) -> ()
                      }
                    }
                  }
                  frame 4 {
                    n647 = stacked-sequence {
                      frame #0 {
                        n648 = local write "Meter SLPM"(50) -> ()
                        n649 = local write "Gas Type"("NG") -> ()
                        n650 = local write "Signal 2"(TRUE) -> ()
                      }
                      frame #1 {
                        n651 = local read "Gas Type"() -> (w701:string)
                        n652 = case shown="\"NG\", Default" w701 {
                          tunnel: [w723 w732] -> w700
                          tunnel: [TRUE FALSE] -> w699
                          tunnel: [FALSE TRUE] -> w698
                          tunnel: [1.0 0.995] -> w697
                          tunnel: [w717 w727] -> w696
                          frame "LP" {
                            n653 = local read "Meter SLPM"() -> (w725:dbl)
                            n654 = Divide(x=w725, y=0.5) -> (x/y=w718:dbl)
                            n655 = Multiply(x=0.211888, y=w718) -> (x*y=w723:dbl)
                            n656 = local read "HeatingValueLP"() -> (w717:dbl)
                            n657 = Multiply(x=w718, y=2600) -> ()  [unwired: 1 out]
                          }
                          frame "NG", Default {
                            n658 = local read "Meter SLPM"() -> (w734:dbl)
                            n659 = Divide(x=w734, y=1.0) -> (x/y=w728:dbl)
                            n660 = Multiply(x=0.423776, y=w728) -> (x*y=w732:dbl)
                            n661 = local read "HeatingValueNG"() -> (w727:dbl)
                          }
                        }
                        n662 = local read "Reference4"() -> (w704:dbl)
                        n663 = local read "Output 4"() -> (w705:dbl)
                        n664 = Divide(x=w705, y=w704) -> (x/y=w702:dbl)
                        n665 = Compound Arithmetic op=MULTIPLY(w702, 5.0, w700) -> (w695:dbl)
                        n666 = local write "CF HR"(w695) -> ()
                        n667 = Divide(x=w695, y=3600) -> (x/y=w693:dbl)
                        n668 = local read "CF HR"() -> (w706:dbl)
                        n669 = local read "HV"() -> (w707:dbl)
                        n670 = Multiply(x=0.025, y=w693) -> (x*y=w690:dbl)
                        n671 = local write "HV"(w696) -> ()
                        n672 = Multiply(x=w706, y=w707) -> (x*y=w708:dbl)
                        n673 = local read "Cubic Ft. Flowed"() -> (w691:dbl)
                        n674 = property on="HeatingValueNG" class="DigNum (strict)"("Visible"=w698) -> ()  [unwired: 2 in, 2 out]
                        n675 = property on="HeatingValueLP" class="DigNum (strict)"("Visible"=w699) -> ()  [unwired: 2 in, 2 out]
                        n676 = Multiply(x=w708, y=w697) -> (x*y=w709:dbl)
                        n677 = Add(x=w690, y=w691) -> (x+y=w689:dbl)
                        n678 = local write "Flow Rate"(w709) -> ()
                        n679 = stacked-sequence {
                          frame #0 {
                            n680 = local read "Sum Time"() -> (w712:dbl)
                            n681 = local read "Data Sampling Rate (s)"() -> (w711:dbl)
                            n682 = Add(x=w712, y=w711) -> (x+y=w710:dbl)
                            n683 = local write "25%RateTime"(w710) -> ()
                            n684 = local write "Sum Time"(w710) -> ()
                          }
                          frame #1 {
                            n685 = local read "Sum Time"() -> (w716:dbl)
                            n686 = Quotient & Remainder(x=w716, y=60) -> (x-y*floor(x/y)=w713:dbl, floor(x/y)=w714:dbl)
                            n687 = local write "Minutes"(w714) -> ()
                            n688 = local write "Seconds"(w713) -> ()
                          }
                        }
                        n689 = local write "Cubic Ft. Flowed"(w689) -> ()
                      }
                    }
                  }
                  frame 5 {
                    n690 = stacked-sequence {
                      frame #0 {
                        n691 = local write "Meter SLPM"(10) -> ()
                        n692 = local write "Gas Type"("LP") -> ()
                        n693 = local write "Signal 2"(TRUE) -> ()
                      }
                      frame #1 {
                        n694 = local read "Gas Type"() -> (w751:string)
                        n695 = case shown="\"NG\", Default" w751 {
                          tunnel: [w773 w782] -> w750
                          tunnel: [TRUE FALSE] -> w749
                          tunnel: [FALSE TRUE] -> w748
                          tunnel: [1.0 0.995] -> w747
                          tunnel: [w767 w777] -> w746
                          frame "LP" {
                            n696 = local read "Meter SLPM"() -> (w775:dbl)
                            n697 = Divide(x=w775, y=0.5) -> (x/y=w768:dbl)
                            n698 = Multiply(x=0.211888, y=w768) -> (x*y=w773:dbl)
                            n699 = local read "HeatingValueLP"() -> (w767:dbl)
                            n700 = Multiply(x=w768, y=2600) -> ()  [unwired: 1 out]
                          }
                          frame "NG", Default {
                            n701 = local read "Meter SLPM"() -> (w784:dbl)
                            n702 = Divide(x=w784, y=1.0) -> (x/y=w778:dbl)
                            n703 = Multiply(x=0.423776, y=w778) -> (x*y=w782:dbl)
                            n704 = local read "HeatingValueNG"() -> (w777:dbl)
                          }
                        }
                        n705 = local read "Reference5"() -> (w754:dbl)
                        n706 = local read "Output 5"() -> (w755:dbl)
                        n707 = Divide(x=w755, y=w754) -> (x/y=w752:dbl)
                        n708 = Compound Arithmetic op=MULTIPLY(w752, 5.0, w750) -> (w745:dbl)
                        n709 = local write "CF HR"(w745) -> ()
                        n710 = Divide(x=w745, y=3600) -> (x/y=w743:dbl)
                        n711 = local read "CF HR"() -> (w756:dbl)
                        n712 = local read "HV"() -> (w757:dbl)
                        n713 = Multiply(x=0.025, y=w743) -> (x*y=w740:dbl)
                        n714 = local write "HV"(w746) -> ()
                        n715 = Multiply(x=w756, y=w757) -> (x*y=w758:dbl)
                        n716 = local read "Cubic Ft. Flowed"() -> (w741:dbl)
                        n717 = property on="HeatingValueNG" class="DigNum (strict)"("Visible"=w748) -> ()  [unwired: 2 in, 2 out]
                        n718 = property on="HeatingValueLP" class="DigNum (strict)"("Visible"=w749) -> ()  [unwired: 2 in, 2 out]
                        n719 = Multiply(x=w758, y=w747) -> (x*y=w759:dbl)
                        n720 = Add(x=w740, y=w741) -> (x+y=w739:dbl)
                        n721 = local write "Flow Rate"(w759) -> ()
                        n722 = stacked-sequence {
                          frame #0 {
                            n723 = local read "Sum Time"() -> (w762:dbl)
                            n724 = local read "Data Sampling Rate (s)"() -> (w761:dbl)
                            n725 = Add(x=w762, y=w761) -> (x+y=w760:dbl)
                            n726 = local write "25%RateTime"(w760) -> ()
                            n727 = local write "Sum Time"(w760) -> ()
                          }
                          frame #1 {
                            n728 = local read "Sum Time"() -> (w766:dbl)
                            n729 = Quotient & Remainder(x=w766, y=60) -> (x-y*floor(x/y)=w763:dbl, floor(x/y)=w764:dbl)
                            n730 = local write "Minutes"(w764) -> ()
                            n731 = local write "Seconds"(w763) -> ()
                          }
                        }
                        n732 = local write "Cubic Ft. Flowed"(w739) -> ()
                      }
                    }
                  }
                  frame 6 {
                    n733 = stacked-sequence {
                      frame #0 {
                        n734 = local write "Meter SLPM"(20) -> ()
                        n735 = local write "Gas Type"("LP") -> ()
                        n736 = local write "Signal 2"(TRUE) -> ()
                      }
                      frame #1 {
                        n737 = local read "Gas Type"() -> (w801:string)
                        n738 = case shown="\"NG\", Default" w801 {
                          tunnel: [w823 w832] -> w800
                          tunnel: [TRUE FALSE] -> w799
                          tunnel: [FALSE TRUE] -> w798
                          tunnel: [1.0 0.995] -> w797
                          tunnel: [w817 w827] -> w796
                          frame "LP" {
                            n739 = local read "Meter SLPM"() -> (w825:dbl)
                            n740 = Divide(x=w825, y=0.5) -> (x/y=w818:dbl)
                            n741 = Multiply(x=0.211888, y=w818) -> (x*y=w823:dbl)
                            n742 = local read "HeatingValueLP"() -> (w817:dbl)
                            n743 = Multiply(x=w818, y=2600) -> ()  [unwired: 1 out]
                          }
                          frame "NG", Default {
                            n744 = local read "Meter SLPM"() -> (w834:dbl)
                            n745 = Divide(x=w834, y=1.0) -> (x/y=w828:dbl)
                            n746 = Multiply(x=0.423776, y=w828) -> (x*y=w832:dbl)
                            n747 = local read "HeatingValueNG"() -> (w827:dbl)
                          }
                        }
                        n748 = local read "Reference6"() -> (w804:dbl)
                        n749 = local read "Output 6"() -> (w805:dbl)
                        n750 = Divide(x=w805, y=w804) -> (x/y=w802:dbl)
                        n751 = Compound Arithmetic op=MULTIPLY(w802, 5.0, w800) -> (w795:dbl)
                        n752 = local write "CF HR"(w795) -> ()
                        n753 = Divide(x=w795, y=3600) -> (x/y=w793:dbl)
                        n754 = local read "CF HR"() -> (w806:dbl)
                        n755 = local read "HV"() -> (w807:dbl)
                        n756 = Multiply(x=0.025, y=w793) -> (x*y=w790:dbl)
                        n757 = local write "HV"(w796) -> ()
                        n758 = Multiply(x=w806, y=w807) -> (x*y=w808:dbl)
                        n759 = local read "Cubic Ft. Flowed"() -> (w791:dbl)
                        n760 = property on="HeatingValueNG" class="DigNum (strict)"("Visible"=w798) -> ()  [unwired: 2 in, 2 out]
                        n761 = property on="HeatingValueLP" class="DigNum (strict)"("Visible"=w799) -> ()  [unwired: 2 in, 2 out]
                        n762 = Multiply(x=w808, y=w797) -> (x*y=w809:dbl)
                        n763 = Add(x=w790, y=w791) -> (x+y=w789:dbl)
                        n764 = stacked-sequence {
                          frame #0 {
                            n765 = local read "Data Sampling Rate (s)"() -> (w811:dbl)
                            n766 = local read "Sum Time"() -> (w812:dbl)
                            n767 = Add(x=w812, y=w811) -> (x+y=w810:dbl)
                            n768 = local write "25%RateTime"(w810) -> ()
                            n769 = local write "Sum Time"(w810) -> ()
                          }
                          frame #1 {
                            n770 = local read "Sum Time"() -> (w816:dbl)
                            n771 = Quotient & Remainder(x=w816, y=60) -> (x-y*floor(x/y)=w813:dbl, floor(x/y)=w814:dbl)
                            n772 = local write "Minutes"(w814) -> ()
                            n773 = local write "Seconds"(w813) -> ()
                          }
                        }
                        n774 = local write "Flow Rate"(w809) -> ()
                        n775 = local write "Cubic Ft. Flowed"(w789) -> ()
                      }
                    }
                  }
                }
              }
              frame #1 {
                n776 = local read "25%Sum"() -> (w844:dbl)
                n777 = local read "Flow Rate"() -> (w845:dbl)
                n778 = local read "25%RateTime"() -> (w841:dbl)
                n779 = Add(x=w845, y=w844) -> (x+y=w843:dbl)
                n780 = Divide(x=w843, y=w841) -> (x/y=w842:dbl)
                n781 = Subtract(x=900.0, y=w841) -> (x-y=w838:dbl)
                n782 = Quotient & Remainder(x=w838, y=60) -> (x-y*floor(x/y)=w836:dbl, floor(x/y)=w837:dbl)
                n783 = local write "Minute"(w837) -> ()
                n784 = local write "25% Rate Run Average"(w842) -> ()
                n785 = local write "Second"(w836) -> ()
              }
            }
            n786 = case shown="True" w504 {
              frame True {
                w518 = refnum<k21> "ReadNGFlowMeterIn"  # DAQmx Task Name
                n787 = call-poly <vilib>:"DAQmx Read.vi"("task/channels in"=w518) -> ("data"=w509:dbl[])  [unwired: 12 in, 2 out]
                n788 = Index Array(array=w509, index=0) -> (element=w514:dbl)
                n789 = Index Array(array=w509, index=1) -> (element=w515:dbl)
                n790 = Index Array(array=w509, index=2) -> (element=w508:dbl)
                n791 = Index Array(array=w509, index=3) -> (element=w507:dbl)
                n792 = Index Array(array=w509, index=4) -> (element=w506:dbl)
                n793 = Index Array(array=w509, index=5) -> (element=w505:dbl)
                n794 = local write "Reference1"(w514) -> ()
                n795 = local write "Reference2"(w515) -> ()
                n796 = local write "Reference3"(w508) -> ()
                n797 = local write "Output 2"(w506) -> ()
                n798 = local write "Output 1"(w507) -> ()
                n799 = local write "Output 3"(w505) -> ()
              }
              frame False {
                w532 = refnum<k21> "ReadLPFlowMeterIn"  # DAQmx Task Name
                n800 = call-poly <vilib>:"DAQmx Read.vi"("task/channels in"=w532) -> ("data"=w523:dbl[])  [unwired: 12 in, 2 out]
                n801 = Index Array(array=w523, index=0) -> (element=w528:dbl)
                n802 = Index Array(array=w523, index=1) -> (element=w529:dbl)
                n803 = Index Array(array=w523, index=2) -> (element=w522:dbl)
                n804 = Index Array(array=w523, index=3) -> (element=w521:dbl)
                n805 = Index Array(array=w523, index=4) -> (element=w520:dbl)
                n806 = Index Array(array=w523, index=5) -> (element=w519:dbl)
                n807 = local write "Reference4"(w528) -> ()
                n808 = local write "Reference5"(w529) -> ()
                n809 = local write "Reference6"(w522) -> ()
                n810 = local write "Output 2"(w520) -> ()
                n811 = local write "Output 1"(w521) -> ()
                n812 = local write "Output 3"(w519) -> ()
              }
            }
          }
        }
      }
    }
    frame "Complete" {
      n813 = while {
        stop <- TRUE continue-if-true
        w878 = FALSE
        n814 = local read "Output 1"() -> (w882:dbl)
        n815 = local read "Reset"() -> (w884:bool)
        n816 = Greater?(x=w882, y=0.1) -> (0:w881:bool)
        n817 = case shown="False" w881 {
          frame False {
            n818 = local read "Output 2"() -> (w1219:dbl)
            n819 = Greater?(x=w1219, y=0.1) -> (0:w1218:bool)
            n820 = case shown="False" w1218 {
              frame False {
                n821 = local read "Output 3"() -> (w1222:dbl)
                n822 = Greater?(x=w1222, y=0.1) -> (0:w1221:bool)
                n823 = case shown="False" w1221 {
                  frame False {
                    n824 = local read "Output 4"() -> (w1226:dbl)
                    n825 = Greater?(x=w1226, y=0.1) -> (0:w1224:bool)
                    n826 = case shown="False" w1224 {
                      frame False {
                        n827 = local read "Output 5"() -> (w1229:dbl)
                        n828 = Greater?(x=w1229, y=0.1) -> (0:w1227:bool)
                        n829 = case shown="False" w1227 {
                          frame False {
                            n830 = local read "Output 6"() -> (w1231:dbl)
                            n831 = Greater?(x=w1231, y=0.1) -> (0:w1230:bool)
                            n832 = case shown="False" w1230 {
                              frame True {
                                n833 = local write "Current Meter"(6.0) -> ()
                                n834 = local write "Signal 2"(TRUE) -> ()
                              }
                              frame False {
                                n835 = local write "Current Meter"(0) -> ()
                                n836 = local write "CurrentState"("Standby") -> ()
                                n837 = local write "Signal 2"(FALSE) -> ()
                              }
                            }
                          }
                          frame True {
                            n838 = local write "Current Meter"(5.0) -> ()
                            n839 = local write "Signal 2"(TRUE) -> ()
                          }
                        }
                      }
                      frame True {
                        n840 = local write "Current Meter"(4.0) -> ()
                        n841 = local write "Signal 2"(TRUE) -> ()
                      }
                    }
                  }
                  frame True {
                    n842 = local write "Current Meter"(3) -> ()
                    n843 = local write "Signal 2"(TRUE) -> ()
                  }
                }
              }
              frame True {
                n844 = local write "Current Meter"(2) -> ()
                n845 = local write "Signal 2"(TRUE) -> ()
              }
            }
          }
          frame True {
            n846 = local write "Current Meter"(1) -> ()
            n847 = local write "Signal 2"(TRUE) -> ()
          }
        }
        n848 = case shown="True" w884 {
          frame False {
          }
          frame True {
            w1249 = 0
            n849 = local write "Cubic Ft. Flowed"(w1249) -> ()
            n850 = local write "Sum Time"(w1249) -> ()
            n851 = local write "Seconds"(w1249) -> ()
            n852 = local write "Minutes"(w1249) -> ()
            n853 = local write "CurrentState"("Standby") -> ()
          }
        }
        n854 = local write "25PercentInRange"(w878) -> ()
        n855 = local write "25PercentRate"(w878) -> ()
        n856 = local write "MaxRateState"(w878) -> ()
        n857 = local read "Data Sampling Rate (s)"() -> (w879:dbl)
        n858 = call "Elapsed Time4"("Time Target (s)"=w879) -> ("Time has Elapsed"=w880:bool)  [unwired: 11 in, 7 out]
        n859 = case shown="True" w880 {
          frame False {
          }
          frame True {
            n860 = stacked-sequence {
              frame #0 {
                n861 = local read "Current Meter"() -> (w915:dbl)
                n862 = case shown="1" w915 {
                  frame 0, Default {
                    n863 = local write "Flow Rate"(0.0) -> ()
                    n864 = local write "Signal 2"(FALSE) -> ()
                  }
                  frame 1 {
                    n865 = stacked-sequence {
                      frame #0 {
                        n866 = local write "Meter SLPM"(1) -> ()
                        n867 = local write "Gas Type"("NG") -> ()
                        n868 = local write "Signal 2"(TRUE) -> ()
                      }
                      frame #1 {
                        n869 = local read "Gas Type"() -> (w933:string)
                        n870 = case shown="\"NG\", Default" w933 {
                          tunnel: [w955 w964] -> w932
                          tunnel: [TRUE FALSE] -> w931
                          tunnel: [FALSE TRUE] -> w930
                          tunnel: [1.0 0.995] -> w929
                          tunnel: [w949 w959] -> w928
                          frame "LP" {
                            n871 = local read "Meter SLPM"() -> (w957:dbl)
                            n872 = Divide(x=w957, y=0.5) -> (x/y=w950:dbl)
                            n873 = Multiply(x=0.211888, y=w950) -> (x*y=w955:dbl)
                            n874 = local read "HeatingValueLP"() -> (w949:dbl)
                            n875 = Multiply(x=w950, y=2600) -> ()  [unwired: 1 out]
                          }
                          frame "NG", Default {
                            n876 = local read "Meter SLPM"() -> (w966:dbl)
                            n877 = Divide(x=w966, y=1.0) -> (x/y=w960:dbl)
                            n878 = Multiply(x=0.423776, y=w960) -> (x*y=w964:dbl)
                            n879 = local read "HeatingValueNG"() -> (w959:dbl)
                          }
                        }
                        n880 = local read "Reference1"() -> (w936:dbl)
                        n881 = local read "Output 1"() -> (w937:dbl)
                        n882 = Divide(x=w937, y=w936) -> (x/y=w934:dbl)
                        n883 = Compound Arithmetic op=MULTIPLY(w934, 5.0, w932) -> (w927:dbl)
                        n884 = local write "CF HR"(w927) -> ()
                        n885 = Divide(x=w927, y=3600) -> (x/y=w925:dbl)
                        n886 = local read "HV"() -> (w939:dbl)
                        n887 = local read "CF HR"() -> (w938:dbl)
                        n888 = local write "HV"(w928) -> ()
                        n889 = Multiply(x=0.025, y=w925) -> (x*y=w922:dbl)
                        n890 = Multiply(x=w938, y=w939) -> (x*y=w940:dbl)
                        n891 = local read "Cubic Ft. Flowed"() -> (w923:dbl)
                        n892 = property on="HeatingValueNG" class="DigNum (strict)"("Visible"=w930) -> ()  [unwired: 2 in, 2 out]
                        n893 = property on="HeatingValueLP" class="DigNum (strict)"("Visible"=w931) -> ()  [unwired: 2 in, 2 out]
                        n894 = Multiply(x=w940, y=w929) -> (x*y=w941:dbl)
                        n895 = Add(x=w922, y=w923) -> (x+y=w921:dbl)
                        n896 = stacked-sequence {
                          frame #0 {
                            n897 = local read "Data Sampling Rate (s)"() -> (w943:dbl)
                            n898 = local read "Sum Time"() -> (w944:dbl)
                            n899 = Add(x=w944, y=w943) -> (x+y=w942:dbl)
                            n900 = local write "25%RateTime"(w942) -> ()
                            n901 = local write "Sum Time"(w942) -> ()
                          }
                          frame #1 {
                            n902 = local read "Sum Time"() -> (w948:dbl)
                            n903 = Quotient & Remainder(x=w948, y=60) -> (x-y*floor(x/y)=w945:dbl, floor(x/y)=w946:dbl)
                            n904 = local write "Minutes"(w946) -> ()
                            n905 = local write "Seconds"(w945) -> ()
                          }
                        }
                        n906 = local write "Flow Rate"(w941) -> ()
                        n907 = local write "Cubic Ft. Flowed"(w921) -> ()
                      }
                    }
                  }
                  frame 2 {
                    n908 = stacked-sequence {
                      frame #0 {
                        n909 = local write "Meter SLPM"(10) -> ()
                        n910 = local write "Gas Type"("NG") -> ()
                        n911 = local write "Signal 2"(TRUE) -> ()
                      }
                      frame #1 {
                        n912 = local read "Gas Type"() -> (w983:string)
                        n913 = case shown="\"NG\", Default" w983 {
                          tunnel: [w1005 w1014] -> w982
                          tunnel: [TRUE FALSE] -> w981
                          tunnel: [FALSE TRUE] -> w980
                          tunnel: [1.0 0.995] -> w979
                          tunnel: [w999 w1009] -> w978
                          frame "LP" {
                            n914 = local read "Meter SLPM"() -> (w1007:dbl)
                            n915 = Divide(x=w1007, y=0.5) -> (x/y=w1000:dbl)
                            n916 = Multiply(x=0.211888, y=w1000) -> (x*y=w1005:dbl)
                            n917 = local read "HeatingValueLP"() -> (w999:dbl)
                            n918 = Multiply(x=w1000, y=2600) -> ()  [unwired: 1 out]
                          }
                          frame "NG", Default {
                            n919 = local read "Meter SLPM"() -> (w1016:dbl)
                            n920 = Divide(x=w1016, y=1.0) -> (x/y=w1010:dbl)
                            n921 = Multiply(x=0.423776, y=w1010) -> (x*y=w1014:dbl)
                            n922 = local read "HeatingValueNG"() -> (w1009:dbl)
                          }
                        }
                        n923 = local read "Reference2"() -> (w986:dbl)
                        n924 = local read "Output 2"() -> (w987:dbl)
                        n925 = Divide(x=w987, y=w986) -> (x/y=w984:dbl)
                        n926 = Compound Arithmetic op=MULTIPLY(w984, 5.0, w982) -> (w977:dbl)
                        n927 = local write "CF HR"(w977) -> ()
                        n928 = Divide(x=w977, y=3600) -> (x/y=w975:dbl)
                        n929 = local read "CF HR"() -> (w988:dbl)
                        n930 = local read "HV"() -> (w989:dbl)
                        n931 = Multiply(x=0.025, y=w975) -> (x*y=w972:dbl)
                        n932 = local write "HV"(w978) -> ()
                        n933 = Multiply(x=w988, y=w989) -> (x*y=w990:dbl)
                        n934 = local read "Cubic Ft. Flowed"() -> (w973:dbl)
                        n935 = property on="HeatingValueNG" class="DigNum (strict)"("Visible"=w980) -> ()  [unwired: 2 in, 2 out]
                        n936 = property on="HeatingValueLP" class="DigNum (strict)"("Visible"=w981) -> ()  [unwired: 2 in, 2 out]
                        n937 = Multiply(x=w990, y=w979) -> (x*y=w991:dbl)
                        n938 = Add(x=w972, y=w973) -> (x+y=w971:dbl)
                        n939 = local write "Flow Rate"(w991) -> ()
                        n940 = stacked-sequence {
                          frame #0 {
                            n941 = local read "Sum Time"() -> (w994:dbl)
                            n942 = local read "Data Sampling Rate (s)"() -> (w993:dbl)
                            n943 = Add(x=w994, y=w993) -> (x+y=w992:dbl)
                            n944 = local write "25%RateTime"(w992) -> ()
                            n945 = local write "Sum Time"(w992) -> ()
                          }
                          frame #1 {
                            n946 = local read "Sum Time"() -> (w998:dbl)
                            n947 = Quotient & Remainder(x=w998, y=60) -> (x-y*floor(x/y)=w995:dbl, floor(x/y)=w996:dbl)
                            n948 = local write "Minutes"(w996) -> ()
                            n949 = local write "Seconds"(w995) -> ()
                          }
                        }
                        n950 = local write "Cubic Ft. Flowed"(w971) -> ()
                      }
                    }
                  }
                  frame 3 {
                    n951 = stacked-sequence {
                      frame #0 {
                        n952 = local write "Meter SLPM"(20) -> ()
                        n953 = local write "Gas Type"("NG") -> ()
                        n954 = local write "Signal 2"(TRUE) -> ()
                      }
                      frame #1 {
                        n955 = local read "Gas Type"() -> (w1033:string)
                        n956 = case shown="\"NG\", Default" w1033 {
                          tunnel: [w1055 w1064] -> w1032
                          tunnel: [TRUE FALSE] -> w1031
                          tunnel: [FALSE TRUE] -> w1030
                          tunnel: [1.0 0.995] -> w1029
                          tunnel: [w1049 w1059] -> w1028
                          frame "LP" {
                            n957 = local read "Meter SLPM"() -> (w1057:dbl)
                            n958 = Divide(x=w1057, y=0.5) -> (x/y=w1050:dbl)
                            n959 = Multiply(x=0.211888, y=w1050) -> (x*y=w1055:dbl)
                            n960 = local read "HeatingValueLP"() -> (w1049:dbl)
                            n961 = Multiply(x=w1050, y=2600) -> ()  [unwired: 1 out]
                          }
                          frame "NG", Default {
                            n962 = local read "Meter SLPM"() -> (w1066:dbl)
                            n963 = Divide(x=w1066, y=1.0) -> (x/y=w1060:dbl)
                            n964 = Multiply(x=0.423776, y=w1060) -> (x*y=w1064:dbl)
                            n965 = local read "HeatingValueNG"() -> (w1059:dbl)
                          }
                        }
                        n966 = local read "Reference3"() -> (w1036:dbl)
                        n967 = local read "Output 3"() -> (w1037:dbl)
                        n968 = Divide(x=w1037, y=w1036) -> (x/y=w1034:dbl)
                        n969 = Compound Arithmetic op=MULTIPLY(w1034, 5.0, w1032) -> (w1027:dbl)
                        n970 = local write "CF HR"(w1027) -> ()
                        n971 = Divide(x=w1027, y=3600) -> (x/y=w1025:dbl)
                        n972 = local read "CF HR"() -> (w1038:dbl)
                        n973 = local read "HV"() -> (w1039:dbl)
                        n974 = Multiply(x=0.025, y=w1025) -> (x*y=w1022:dbl)
                        n975 = local write "HV"(w1028) -> ()
                        n976 = Multiply(x=w1038, y=w1039) -> (x*y=w1040:dbl)
                        n977 = local read "Cubic Ft. Flowed"() -> (w1023:dbl)
                        n978 = property on="HeatingValueNG" class="DigNum (strict)"("Visible"=w1030) -> ()  [unwired: 2 in, 2 out]
                        n979 = property on="HeatingValueLP" class="DigNum (strict)"("Visible"=w1031) -> ()  [unwired: 2 in, 2 out]
                        n980 = Multiply(x=w1040, y=w1029) -> (x*y=w1041:dbl)
                        n981 = Add(x=w1022, y=w1023) -> (x+y=w1021:dbl)
                        n982 = local write "Flow Rate"(w1041) -> ()
                        n983 = stacked-sequence {
                          frame #0 {
                            n984 = local read "Data Sampling Rate (s)"() -> (w1043:dbl)
                            n985 = local read "Sum Time"() -> (w1044:dbl)
                            n986 = Add(x=w1044, y=w1043) -> (x+y=w1042:dbl)
                            n987 = local write "25%RateTime"(w1042) -> ()
                            n988 = local write "Sum Time"(w1042) -> ()
                          }
                          frame #1 {
                            n989 = local read "Sum Time"() -> (w1048:dbl)
                            n990 = Quotient & Remainder(x=w1048, y=60) -> (x-y*floor(x/y)=w1045:dbl, floor(x/y)=w1046:dbl)
                            n991 = local write "Minutes"(w1046) -> ()
                            n992 = local write "Seconds"(w1045) -> ()
                          }
                        }
                        n993 = local write "Cubic Ft. Flowed"(w1021) -> ()
                      }
                    }
                  }
                  frame 4 {
                    n994 = stacked-sequence {
                      frame #0 {
                        n995 = local write "Meter SLPM"(50) -> ()
                        n996 = local write "Gas Type"("NG") -> ()
                        n997 = local write "Signal 2"(TRUE) -> ()
                      }
                      frame #1 {
                        n998 = local read "Gas Type"() -> (w1083:string)
                        n999 = case shown="\"NG\", Default" w1083 {
                          tunnel: [w1105 w1114] -> w1082
                          tunnel: [TRUE FALSE] -> w1081
                          tunnel: [FALSE TRUE] -> w1080
                          tunnel: [1.0 0.995] -> w1079
                          tunnel: [w1099 w1109] -> w1078
                          frame "LP" {
                            n1000 = local read "Meter SLPM"() -> (w1107:dbl)
                            n1001 = Divide(x=w1107, y=0.5) -> (x/y=w1100:dbl)
                            n1002 = Multiply(x=0.211888, y=w1100) -> (x*y=w1105:dbl)
                            n1003 = local read "HeatingValueLP"() -> (w1099:dbl)
                            n1004 = Multiply(x=w1100, y=2600) -> ()  [unwired: 1 out]
                          }
                          frame "NG", Default {
                            n1005 = local read "Meter SLPM"() -> (w1116:dbl)
                            n1006 = Divide(x=w1116, y=1.0) -> (x/y=w1110:dbl)
                            n1007 = Multiply(x=0.423776, y=w1110) -> (x*y=w1114:dbl)
                            n1008 = local read "HeatingValueNG"() -> (w1109:dbl)
                          }
                        }
                        n1009 = local read "Reference4"() -> (w1086:dbl)
                        n1010 = local read "Output 4"() -> (w1087:dbl)
                        n1011 = Divide(x=w1087, y=w1086) -> (x/y=w1084:dbl)
                        n1012 = Compound Arithmetic op=MULTIPLY(w1084, 5.0, w1082) -> (w1077:dbl)
                        n1013 = local write "CF HR"(w1077) -> ()
                        n1014 = Divide(x=w1077, y=3600) -> (x/y=w1075:dbl)
                        n1015 = local read "CF HR"() -> (w1088:dbl)
                        n1016 = local read "HV"() -> (w1089:dbl)
                        n1017 = Multiply(x=0.025, y=w1075) -> (x*y=w1072:dbl)
                        n1018 = local write "HV"(w1078) -> ()
                        n1019 = Multiply(x=w1088, y=w1089) -> (x*y=w1090:dbl)
                        n1020 = local read "Cubic Ft. Flowed"() -> (w1073:dbl)
                        n1021 = property on="HeatingValueNG" class="DigNum (strict)"("Visible"=w1080) -> ()  [unwired: 2 in, 2 out]
                        n1022 = property on="HeatingValueLP" class="DigNum (strict)"("Visible"=w1081) -> ()  [unwired: 2 in, 2 out]
                        n1023 = Multiply(x=w1090, y=w1079) -> (x*y=w1091:dbl)
                        n1024 = Add(x=w1072, y=w1073) -> (x+y=w1071:dbl)
                        n1025 = local write "Flow Rate"(w1091) -> ()
                        n1026 = stacked-sequence {
                          frame #0 {
                            n1027 = local read "Sum Time"() -> (w1094:dbl)
                            n1028 = local read "Data Sampling Rate (s)"() -> (w1093:dbl)
                            n1029 = Add(x=w1094, y=w1093) -> (x+y=w1092:dbl)
                            n1030 = local write "25%RateTime"(w1092) -> ()
                            n1031 = local write "Sum Time"(w1092) -> ()
                          }
                          frame #1 {
                            n1032 = local read "Sum Time"() -> (w1098:dbl)
                            n1033 = Quotient & Remainder(x=w1098, y=60) -> (x-y*floor(x/y)=w1095:dbl, floor(x/y)=w1096:dbl)
                            n1034 = local write "Minutes"(w1096) -> ()
                            n1035 = local write "Seconds"(w1095) -> ()
                          }
                        }
                        n1036 = local write "Cubic Ft. Flowed"(w1071) -> ()
                      }
                    }
                  }
                  frame 5 {
                    n1037 = stacked-sequence {
                      frame #0 {
                        n1038 = local write "Meter SLPM"(10) -> ()
                        n1039 = local write "Gas Type"("LP") -> ()
                        n1040 = local write "Signal 2"(TRUE) -> ()
                      }
                      frame #1 {
                        n1041 = local read "Gas Type"() -> (w1133:string)
                        n1042 = case shown="\"NG\", Default" w1133 {
                          tunnel: [w1155 w1164] -> w1132
                          tunnel: [TRUE FALSE] -> w1131
                          tunnel: [FALSE TRUE] -> w1130
                          tunnel: [1.0 0.995] -> w1129
                          tunnel: [w1149 w1159] -> w1128
                          frame "LP" {
                            n1043 = local read "Meter SLPM"() -> (w1157:dbl)
                            n1044 = Divide(x=w1157, y=0.5) -> (x/y=w1150:dbl)
                            n1045 = Multiply(x=0.211888, y=w1150) -> (x*y=w1155:dbl)
                            n1046 = local read "HeatingValueLP"() -> (w1149:dbl)
                            n1047 = Multiply(x=w1150, y=2600) -> ()  [unwired: 1 out]
                          }
                          frame "NG", Default {
                            n1048 = local read "Meter SLPM"() -> (w1166:dbl)
                            n1049 = Divide(x=w1166, y=1.0) -> (x/y=w1160:dbl)
                            n1050 = Multiply(x=0.423776, y=w1160) -> (x*y=w1164:dbl)
                            n1051 = local read "HeatingValueNG"() -> (w1159:dbl)
                          }
                        }
                        n1052 = local read "Reference5"() -> (w1136:dbl)
                        n1053 = local read "Output 5"() -> (w1137:dbl)
                        n1054 = Divide(x=w1137, y=w1136) -> (x/y=w1134:dbl)
                        n1055 = Compound Arithmetic op=MULTIPLY(w1134, 5.0, w1132) -> (w1127:dbl)
                        n1056 = local write "CF HR"(w1127) -> ()
                        n1057 = Divide(x=w1127, y=3600) -> (x/y=w1125:dbl)
                        n1058 = local read "CF HR"() -> (w1138:dbl)
                        n1059 = local read "HV"() -> (w1139:dbl)
                        n1060 = Multiply(x=0.025, y=w1125) -> (x*y=w1122:dbl)
                        n1061 = local write "HV"(w1128) -> ()
                        n1062 = Multiply(x=w1138, y=w1139) -> (x*y=w1140:dbl)
                        n1063 = local read "Cubic Ft. Flowed"() -> (w1123:dbl)
                        n1064 = property on="HeatingValueNG" class="DigNum (strict)"("Visible"=w1130) -> ()  [unwired: 2 in, 2 out]
                        n1065 = property on="HeatingValueLP" class="DigNum (strict)"("Visible"=w1131) -> ()  [unwired: 2 in, 2 out]
                        n1066 = Multiply(x=w1140, y=w1129) -> (x*y=w1141:dbl)
                        n1067 = Add(x=w1122, y=w1123) -> (x+y=w1121:dbl)
                        n1068 = local write "Flow Rate"(w1141) -> ()
                        n1069 = stacked-sequence {
                          frame #0 {
                            n1070 = local read "Sum Time"() -> (w1144:dbl)
                            n1071 = local read "Data Sampling Rate (s)"() -> (w1143:dbl)
                            n1072 = Add(x=w1144, y=w1143) -> (x+y=w1142:dbl)
                            n1073 = local write "25%RateTime"(w1142) -> ()
                            n1074 = local write "Sum Time"(w1142) -> ()
                          }
                          frame #1 {
                            n1075 = local read "Sum Time"() -> (w1148:dbl)
                            n1076 = Quotient & Remainder(x=w1148, y=60) -> (x-y*floor(x/y)=w1145:dbl, floor(x/y)=w1146:dbl)
                            n1077 = local write "Minutes"(w1146) -> ()
                            n1078 = local write "Seconds"(w1145) -> ()
                          }
                        }
                        n1079 = local write "Cubic Ft. Flowed"(w1121) -> ()
                      }
                    }
                  }
                  frame 6 {
                    n1080 = stacked-sequence {
                      frame #0 {
                        n1081 = local write "Meter SLPM"(20) -> ()
                        n1082 = local write "Gas Type"("LP") -> ()
                        n1083 = local write "Signal 2"(TRUE) -> ()
                      }
                      frame #1 {
                        n1084 = local read "Gas Type"() -> (w1183:string)
                        n1085 = case shown="\"NG\", Default" w1183 {
                          tunnel: [w1205 w1214] -> w1182
                          tunnel: [TRUE FALSE] -> w1181
                          tunnel: [FALSE TRUE] -> w1180
                          tunnel: [1.0 0.995] -> w1179
                          tunnel: [w1199 w1209] -> w1178
                          frame "LP" {
                            n1086 = local read "Meter SLPM"() -> (w1207:dbl)
                            n1087 = Divide(x=w1207, y=0.5) -> (x/y=w1200:dbl)
                            n1088 = Multiply(x=0.211888, y=w1200) -> (x*y=w1205:dbl)
                            n1089 = local read "HeatingValueLP"() -> (w1199:dbl)
                            n1090 = Multiply(x=w1200, y=2600) -> ()  [unwired: 1 out]
                          }
                          frame "NG", Default {
                            n1091 = local read "Meter SLPM"() -> (w1216:dbl)
                            n1092 = Divide(x=w1216, y=1.0) -> (x/y=w1210:dbl)
                            n1093 = Multiply(x=0.423776, y=w1210) -> (x*y=w1214:dbl)
                            n1094 = local read "HeatingValueNG"() -> (w1209:dbl)
                          }
                        }
                        n1095 = local read "Reference6"() -> (w1186:dbl)
                        n1096 = local read "Output 6"() -> (w1187:dbl)
                        n1097 = Divide(x=w1187, y=w1186) -> (x/y=w1184:dbl)
                        n1098 = Compound Arithmetic op=MULTIPLY(w1184, 5.0, w1182) -> (w1177:dbl)
                        n1099 = local write "CF HR"(w1177) -> ()
                        n1100 = Divide(x=w1177, y=3600) -> (x/y=w1175:dbl)
                        n1101 = local read "CF HR"() -> (w1188:dbl)
                        n1102 = local read "HV"() -> (w1189:dbl)
                        n1103 = Multiply(x=0.025, y=w1175) -> (x*y=w1172:dbl)
                        n1104 = local write "HV"(w1178) -> ()
                        n1105 = Multiply(x=w1188, y=w1189) -> (x*y=w1190:dbl)
                        n1106 = local read "Cubic Ft. Flowed"() -> (w1173:dbl)
                        n1107 = property on="HeatingValueNG" class="DigNum (strict)"("Visible"=w1180) -> ()  [unwired: 2 in, 2 out]
                        n1108 = property on="HeatingValueLP" class="DigNum (strict)"("Visible"=w1181) -> ()  [unwired: 2 in, 2 out]
                        n1109 = Multiply(x=w1190, y=w1179) -> (x*y=w1191:dbl)
                        n1110 = Add(x=w1172, y=w1173) -> (x+y=w1171:dbl)
                        n1111 = stacked-sequence {
                          frame #0 {
                            n1112 = local read "Data Sampling Rate (s)"() -> (w1193:dbl)
                            n1113 = local read "Sum Time"() -> (w1194:dbl)
                            n1114 = Add(x=w1194, y=w1193) -> (x+y=w1192:dbl)
                            n1115 = local write "25%RateTime"(w1192) -> ()
                            n1116 = local write "Sum Time"(w1192) -> ()
                          }
                          frame #1 {
                            n1117 = local read "Sum Time"() -> (w1198:dbl)
                            n1118 = Quotient & Remainder(x=w1198, y=60) -> (x-y*floor(x/y)=w1195:dbl, floor(x/y)=w1196:dbl)
                            n1119 = local write "Minutes"(w1196) -> ()
                            n1120 = local write "Seconds"(w1195) -> ()
                          }
                        }
                        n1121 = local write "Flow Rate"(w1191) -> ()
                        n1122 = local write "Cubic Ft. Flowed"(w1171) -> ()
                      }
                    }
                  }
                }
              }
            }
            n1123 = local read "NG"() -> (w886:bool)
            n1124 = case shown="True" w886 {
              frame True {
                w900 = refnum<k21> "ReadNGFlowMeterIn"  # DAQmx Task Name
                n1125 = call-poly <vilib>:"DAQmx Read.vi"("task/channels in"=w900) -> ("data"=w891:dbl[])  [unwired: 12 in, 2 out]
                n1126 = Index Array(array=w891, index=0) -> (element=w896:dbl)
                n1127 = Index Array(array=w891, index=1) -> (element=w897:dbl)
                n1128 = Index Array(array=w891, index=2) -> (element=w890:dbl)
                n1129 = Index Array(array=w891, index=3) -> (element=w889:dbl)
                n1130 = Index Array(array=w891, index=4) -> (element=w888:dbl)
                n1131 = Index Array(array=w891, index=5) -> (element=w887:dbl)
                n1132 = local write "Reference1"(w896) -> ()
                n1133 = local write "Reference2"(w897) -> ()
                n1134 = local write "Reference3"(w890) -> ()
                n1135 = local write "Output 2"(w888) -> ()
                n1136 = local write "Output 1"(w889) -> ()
                n1137 = local write "Output 3"(w887) -> ()
              }
              frame False {
                w914 = refnum<k21> "ReadLPFlowMeterIn"  # DAQmx Task Name
                n1138 = call-poly <vilib>:"DAQmx Read.vi"("task/channels in"=w914) -> ("data"=w905:dbl[])  [unwired: 12 in, 2 out]
                n1139 = Index Array(array=w905, index=0) -> (element=w910:dbl)
                n1140 = Index Array(array=w905, index=1) -> (element=w911:dbl)
                n1141 = Index Array(array=w905, index=2) -> (element=w904:dbl)
                n1142 = Index Array(array=w905, index=3) -> (element=w903:dbl)
                n1143 = Index Array(array=w905, index=4) -> (element=w902:dbl)
                n1144 = Index Array(array=w905, index=5) -> (element=w901:dbl)
                n1145 = local write "Reference4"(w910) -> ()
                n1146 = local write "Reference5"(w911) -> ()
                n1147 = local write "Reference6"(w904) -> ()
                n1148 = local write "Output 5"(w902) -> ()
                n1149 = local write "Output 4"(w903) -> ()
                n1150 = local write "Output 6"(w901) -> ()
              }
            }
          }
        }
      }
    }
  }
